vi "4.0.0_Airwatts_Tunings_&_Performance_Test_Max_Power_MODE.vi"(7 "Data in":T1, 8 "error in (no error)":errorcluster, 9 "AllControls In":T2, 10 "?":T3, 11 "Message Queue out":T4) -> (0 "error out":errorcluster, 1 "Flow":string, 2 "Data":T3, 3 "Message Queue Out":T4, 5 "Data out":T1)   [LabVIEW 2017]
uses:
  Depends/AMC/subVIs/TypeDefs/amc_Message Queue.ctl
  Depends/AMC/subVIs/TypeDefs/amc_Message.ctl
  Depends/Tools/Keyed Array/Tools_KeyedArray KeyedArray.ctl
  Ctrls/Data.ctl
  Ctrls/AllControls.ctl
  Ctrls/CSV_Data.ctl
  DIPC 692 Daemon API/typdef/get_parameter.ctl
  DIPC 692 Daemon API/typdef/calibration.ctl
  <vilib>/Analysis/baseanly.llb/Mean (DBL).vi
  Ctrls/AlarmIndex.ctl
  <vilib>/Analysis/NI_AALBase.lvlib
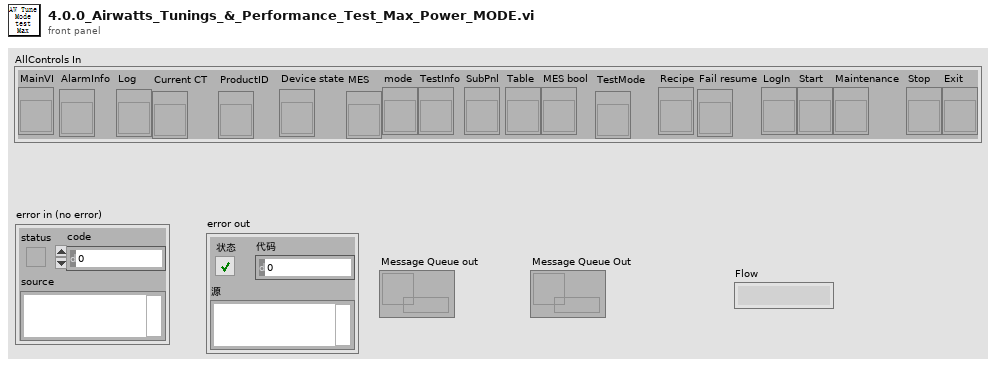
[diagram p1: front panel]
types:
  T1 = typedef "CSV_Data.ctl" = cluster{"Initialisation":cluster{"LMT - Connect UUT (con COM)":string, "LMT - Software Version (rrel)":string, "LMT - Write SKU file (wskuc)":string, "LMT - SKU file name":string, "Connect UUT DDM":string, "Read DDM EOL Timestamp - Mode":string, "Read DDM EOL Timestamp - Timestamp":string, "Read DDM EOL Timestamp - Rig ID":string, "Read DDM EOL Timestamp - Passmark ID":string, "Read DDM EOL Timestamp - Passmark Rev":string, "Software Version before flashing":string, "Read Hardware Serial":string, "UUT DDM SN":string, "Compare DDM SN with MES SN":string, "Backup PCBA Calibration EEPROM Response - CAL":string, "Flash Firmware Version":string, "Check SW Version":string, "Read DDM SW Version after flashing":string, "Set SKU Config":string, "Ready Status":string, "Set Device Mode to EOL":string, "DDM Parameter - Voltage":string, "DDM Parameter - Current":string, "DDM Parameter - Power":string, "DDM Parameter - Speed":string, "DDM Parameter - Pressure":string, "Tester Parameter - Voltage":string, "Tester Parameter - Current":string, "Tester Parameter - Power":string, "Tester Parameter - Ambient Pressure":string, "Tester Parameter - Ambient Temperature":string, "Calculated Parameter - DDM Pressure Corrected":string, "Calculated Parameter - DDM Real Power":string, "Calculated Parameter - Delta V":string}, "BEMF_Calibration":cluster{"Calibration Result - eol_cold_bemf_temp":string, "DDM Ambient Temp":string, "Restriction Plate Diameter":string, "Calibration Result - eol_bemf_mp_cold_coef_a":string, "Calibration Result - eol_bemf_mp_cold_coef_b":string, "Calibration Result - eol_bemf_mp_cold_coef_c":string, "Calibration Result - eol_bemf_lsi_cold_ref_coeffs":string, "Get - Calibration Result - eol_bemf_lsi_speed":string, "Get - Calibration Result - eol_bemf_lsi_integral_0":string, "Calibration Result - eol_bemf_lsi_integral_1":string, "Get - Calibration Result - eol_bemf_lsi_integral_2":string, "Get - Calibration Result - eol_cold_bemf":string, "Get - Calibration Result - eol_cold_bemf_fisf":string, "Finalise Calibration":string, "Compare -Calibration Result - eol_cold_bemf":string, "Compare -Calibration Result - eol_cold_bemf_fisf":string}, "ECO":cluster{"Reset Power Tune":string, "Reset BEMF FISF Calibration":string, "Restriction Plate Diameter":string, "ECO - Stabilisation Time":string, "ECO - DDM Parameter - Voltage":string, "ECO - DDM Parameter - Current":string, "ECO - DDM Parameter - Power":string, "ECO - DDM Parameter - Measured Power":string, "ECO - DDM Parameter - Speed":string, "ECO - DDM Parameter - Pressure":string, "ECO - Tester Parameter - Voltage":string, "ECO - Tester Parameter - Current":string, "ECO - Tester Parameter - Power":string, "ECO - Tester Parameter - Ambient Pressure":string, "ECO - Tester Parameter - Ambient Temperature":string, "ECO - Tester Parameter - Ambient Humidity":string, "ECO - Calculated Parameter - DDM Pressure Corrected":string, "ECO - Calculated Parameter - DDM Real Power":string, "ECO - Calculated Parameter - Delta V":string, "ECO - Calculated Parameter - Flowrate":string, "ECO - Calculated Parameter - Airwatt":string, "ECO - Formula":string, "PT ECO - Power Tune Mode Status":string}, "BOOST":cluster{"Restriction Plate Diameter":string, "BOOST - Stabilisation Time":string, "BOOST - DDM Parameter - Voltage":string, "BOOST - DDM Parameter - Current":string, "BOOST - DDM Parameter - Power":string, "BOOST - DDM Parameter - Measured Power":string, "BOOST - DDM Parameter - Speed":string, "BOOST - DDM Parameter - Pressure":string, "BOOST - Tester Parameter - Voltage":string, "BOOST - Tester Parameter - Current":string, "BOOST - Tester Parameter - Power":string, "BOOST - Tester Parameter - Ambient Pressure":string, "BOOST - Tester Parameter - Ambient Temperature":string, "BOOST - Tester Parameter - Ambient Humidity":string, "BOOST - Calculated Parameter - DDM Pressure Corrected":string, "BOOST - Calculated Parameter - DDM Real Power":string, "BOOST - Calculated Parameter - Delta V":string, "BOOST - Calculated Parameter - Flowrate":string, "BOOST - Calculated Parameter - Airwatt":string, "BOOST - Get AM Presence":string, "Air Muscle Turn Off Status":string, "BOOST - Air Muscle Calculated Parameter - Airwatt B":string, "BOOST - Air Muscle Calculate Airwatt Delta":string, "PT BOOST - Power Tune Mode Status":string, "Finalise Calibration":string, "ECO - Get AW Calibration value":string, "BOOST - Get AW Calibration value":string}, "MAX":cluster{"Restriction Plate Diameter":string, "MAX - Stabilisation Time":string, "Get Average Delta Tmag (LSIdelta_FISFdelta_LSItmag_FISFtmag_IIRtmag)":string, "Get Average Delta Tmag FISF":string, "MAX - DDM Parameter - Voltage":string, "MAX - DDM Parameter - Current":string, "MAX - DDM Parameter - Power":string, "MAX - DDM Parameter - Measured Power":string, "MAX - DDM Parameter - Speed":string, "MAX - DDM Parameter - Pressure":string, "MAX - Tester Parameter - Voltage":string, "MAX - Tester Parameter - Current":string, "MAX - Tester Parameter - Power":string, "MAX - Tester Parameter - Ambient Pressure":string, "MAX - Tester Parameter - Ambient Temperature":string, "MAX - Tester Parameter - Ambient Humidity":string, "MAX - Calculated Parameter - DDM Pressure Corrected":string, "MAX - Calculated Parameter - DDM Real Power":string, "MAX - Calculated Parameter - Delta V":string, "MAX - Calculated Parameter - Flowrate":string, "MAX - Calculated Parameter - Airwatt":string, "MAX_FISF_Check_Average_Delta_Tmag":string, "MAX - FISF - BEMF Finetune Result":string, "MAX tune - Delta P1":string, "MAX tune - Calculated Parameter - Airwatt":string, "Calculate Delta Airwatts - MAX finetune - Delta P2":string, "MAX finetune - DDM Parameter - Voltage":string, "MAX finetune - DDM Parameter - Current":string, "MAX finetune - DDM Parameter - Power":string, "MAX finetune - DDM Parameter - Measured Power":string, "MAX finetune - DDM Parameter - Speed":string, "MAX finetune - DDM Parameter - Pressure":string, "MAX finetune - Tester Parameter - Voltage":string, "MAX finetune - Tester Parameter - Current":string, "MAX finetune - Tester Parameter - Power":string, "MAX finetune - Tester Parameter - Ambient Pressure":string, "MAX finetune - Tester Parameter - Ambient Temperature":string, "MAX finetune - Tester Parameter - Ambient Humidity":string, "MAX finetune - Calculated Parameter - DDM Pressure Corrected":string, "MAX finetune - Calculated Parameter - DDM Real Power":string, "MAX finetune - Calculated Parameter - Delta V":string, "MAX finetune - Calculated Parameter - Flowrate":string, "MAX finetune - Calculated Parameter - Airwatt":string, "Check Derate Result":string, "Delta Tmag FISF":string, "Get Hot BEMF Result":string, "Calculate delta Pressure":string, "Finalise Calibration":string, "Calculate & Check Delta BEMF":string, "Delta P Airwatts Value":string}, "LL":cluster{"DDM Ambient Temp":string, "Restriction Plate Diameter":string, "LL - DDM Parameter - Voltage":string, "LL - DDM Parameter - Current":string, "LL - DDM Parameter - Power":string, "LL - DDM Parameter - Measured Power":string, "LL - DDM Parameter - Speed":string, "LL - DDM Parameter - Pressure":string, "LL - Tester Parameter - Voltage":string, "LL - Tester Parameter - Current":string, "LL - Tester Parameter - Power":string, "LL - DDM Real Power":string, "LL - Calibrate Task Detect LL":string}, "HL":cluster{"HL - DDM Parameter - Voltage":string, "HL - DDM Parameter - Current":string, "HL - DDM Parameter - Power":string, "HL - DDM Parameter - Measured Power":string, "HL - DDM Parameter - Speed":string, "HL - DDM Parameter - Pressure":string, "HL - Tester Parameter - Voltage":string, "HL - Tester Parameter - Current":string, "HL - Tester Parameter - Power":string, "HL - DDM Real Power":string, "HL - Calibrate Task Detect HL":string}, "LH":cluster{"Restriction Plate Diameter":string, "LH - DDM Parameter - Voltage":string, "LH - DDM Parameter - Current":string, "LH - DDM Parameter - Power":string, "LH - DDM Parameter - Measured Power":string, "LH - DDM Parameter - Speed":string, "LH - DDM Parameter - Pressure":string, "LH - Tester Parameter - Voltage":string, "LH - Tester Parameter - Current":string, "LH - Tester Parameter - Power":string, "LH - DDM Real Power":string, "LH - Calibrate Task Detect LH":string}, "HH":cluster{"HH - DDM Parameter - Voltage":string, "HH - DDM Parameter - Current":string, "HH - DDM Parameter - Power":string, "HH - DDM Parameter - Measured Power":string, "HH - DDM Parameter - Speed":string, "HH - DDM Parameter - Pressure":string, "HH - Tester Parameter - Voltage":string, "HH - Tester Parameter - Current":string, "HH - Tester Parameter - Power":string, "HH - DDM Real Power":string, "HH - Calibrate Task Detect HH":string}, "Inlet Blockage Calibration":cluster{"Inlet Blockage Calibration - DDM Parameter - Voltage":string, "Inlet Blockage Calibration - DDM Parameter - Current":string, "Inlet Blockage Calibration - DDM Parameter - Power":string, "Inlet Blockage Calibration - DDM Parameter - Measured Power":string, "Inlet Blockage Calibration - DDM Parameter - Speed":string, "Inlet Blockage Calibration - DDM Parameter - Pressure":string, "Inlet Blockage Calibration - Tester Parameter - Voltage":string, "Inlet Blockage Calibration - Tester Parameter - Current":string, "Inlet Blockage Calibration - Tester Parameter - Power":string, "Inlet Blockage Calibration - DDM Real Power":string, "Calibration Inlet Blockage_E":string, "Finalise Calibration":string, "Get Task Detect LL":string, "Get Task Detect HL":string, "Get Task Detect LH":string, "Get Task Detect HH":string, "Calibration Inlet Blockage":string, "Calibration eol cold bemf temp":string}, "GOOD":cluster{"GOOD UNIT - Clear EEPROM Error Log":string, "GOOD UNIT - Write Product Timestamp - Mode":string, "GOOD UNIT - Write Product Timestamp - Timestamp":string, "GOOD UNIT - Write Product Timestamp - Rig ID":string, "GOOD UNIT - Write Product Timestamp - Passmark ID":string, "GOOD UNIT - Write Product Timestamp - Passmark Rev":string, "GOOD UNIT - Set Device Mode to PROD":string, "GOOD UNIT - Backup PCBA Calibration EEPROM Response":string, "GOOD UNIT - Check Security Bit":string, "GOOD UNIT - Set Calibration Lock":string, "GOOD UNIT - Get_Calibration_Lock":string, "GOOD UNIT - Disconnect UUT":string}, "NG":cluster{"NG UNIT - Read NVM Error":string, "NG UNIT - Set Device Mode to FCT":string, "NG UNIT - Backup PCBA Calibration EEPROM Response - CAL":string, "NG UNIT - Backup PCBA Calibration EEPROM Response - ERROR":string, "NG UNIT - Backup PCBA Calibration EEPROM Response - USAGE":string, "NG UNIT - Disconnect UUT":string}, "SN":string, "Table":string[][], "Count":cluster{"Total":i32, "OK":i32, "NG":i32, "Yield":dbl}, "Start Time":timestamp, "daemon reference":refnum<k5>, "CT":dbl, "Config":string[][], "OK/NG":bool, "Station ID":string, "MES DDM SN":string, "MES PCBA SN":string, "Retest":string, "Lux":string, "Initialisation_Status":cluster{"LMT - Connect UUT (con COM)":string, "LMT - Software Version (rrel)":string, "LMT - Write SKU file (wskuc)":string, "LMT - SKU file name":string, "Connect UUT DDM":string, "Read DDM EOL Timestamp - Mode":string, "Read DDM EOL Timestamp - Timestamp":string, "Read DDM EOL Timestamp - Rig ID":string, "Read DDM EOL Timestamp - Passmark ID":string, "Read DDM EOL Timestamp - Passmark Rev":string, "Software Version before flashing":string, "Read Hardware Serial":string, "UUT DDM SN":string, "Compare DDM SN with MES SN":string, "Backup PCBA Calibration EEPROM Response - CAL":string, "Flash Firmware Version":string, "Check SW Version":string, "Read DDM SW Version after flashing":string, "Set SKU Config":string, "Ready Status":string, "Set Device Mode to EOL":string, "DDM Parameter - Voltage":string, "DDM Parameter - Current":string, "DDM Parameter - Power":string, "DDM Parameter - Speed":string, "DDM Parameter - Pressure":string, "Tester Parameter - Voltage":string, "Tester Parameter - Current":string, "Tester Parameter - Power":string, "Tester Parameter - Ambient Pressure":string, "Tester Parameter - Ambient Temperature":string, "Calculated Parameter - DDM Pressure Corrected":string, "Calculated Parameter - DDM Real Power":string, "Calculated Parameter - Delta V":string}, "BEMF_Calibration_Status":cluster{"Calibration Result - eol_cold_bemf_temp":string, "DDM Ambient Temp":string, "Restriction Plate Diameter":string, "Calibration Result - eol_bemf_mp_cold_coef_a":string, "Calibration Result - eol_bemf_mp_cold_coef_b":string, "Calibration Result - eol_bemf_mp_cold_coef_c":string, "Calibration Result - eol_bemf_lsi_cold_ref_coeffs":string, "Get - Calibration Result - eol_bemf_lsi_speed":string, "Get - Calibration Result - eol_bemf_lsi_integral_0":string, "Calibration Result - eol_bemf_lsi_integral_1":string, "Get - Calibration Result - eol_bemf_lsi_integral_2":string, "Get - Calibration Result - eol_cold_bemf":string, "Get - Calibration Result - eol_cold_bemf_fisf":string, "Finalise Calibration":string, "Compare -Calibration Result - eol_cold_bemf":string, "Compare -Calibration Result - eol_cold_bemf_fisf":string}, "ECO_Status":cluster{"Reset Power Tune":string, "Reset BEMF FISF Calibration":string, "Restriction Plate Diameter":string, "ECO - Stabilisation Time":string, "ECO - DDM Parameter - Voltage":string, "ECO - DDM Parameter - Current":string, "ECO - DDM Parameter - Power":string, "ECO - DDM Parameter - Measured Power":string, "ECO - DDM Parameter - Speed":string, "ECO - DDM Parameter - Pressure":string, "ECO - Tester Parameter - Voltage":string, "ECO - Tester Parameter - Current":string, "ECO - Tester Parameter - Power":string, "ECO - Tester Parameter - Ambient Pressure":string, "ECO - Tester Parameter - Ambient Temperature":string, "ECO - Tester Parameter - Ambient Humidity":string, "ECO - Calculated Parameter - DDM Pressure Corrected":string, "ECO - Calculated Parameter - DDM Real Power":string, "ECO - Calculated Parameter - Delta V":string, "ECO - Calculated Parameter - Flowrate":string, "ECO - Calculated Parameter - Airwatt":string, "ECO - Formula":string, "PT ECO - Power Tune Mode Status":string}, "BOOST_Status":cluster{"Restriction Plate Diameter":string, "BOOST - Stabilisation Time":string, "BOOST - DDM Parameter - Voltage":string, "BOOST - DDM Parameter - Current":string, "BOOST - DDM Parameter - Power":string, "BOOST - DDM Parameter - Measured Power":string, "BOOST - DDM Parameter - Speed":string, "BOOST - DDM Parameter - Pressure":string, "BOOST - Tester Parameter - Voltage":string, "BOOST - Tester Parameter - Current":string, "BOOST - Tester Parameter - Power":string, "BOOST - Tester Parameter - Ambient Pressure":string, "BOOST - Tester Parameter - Ambient Temperature":string, "BOOST - Tester Parameter - Ambient Humidity":string, "BOOST - Calculated Parameter - DDM Pressure Corrected":string, "BOOST - Calculated Parameter - DDM Real Power":string, "BOOST - Calculated Parameter - Delta V":string, "BOOST - Calculated Parameter - Flowrate":string, "BOOST - Calculated Parameter - Airwatt":string, "BOOST - Get AM Presence":string, "Air Muscle Turn Off Status":string, "BOOST - Air Muscle Calculated Parameter - Airwatt B":string, "BOOST - Air Muscle Calculate Airwatt Delta":string, "PT BOOST - Power Tune Mode Status":string, "Finalise Calibration":string, "ECO - Get AW Calibration value":string, "BOOST - Get AW Calibration value":string}, "MAX_Status":cluster{"Restriction Plate Diameter":string, "MAX - Stabilisation Time":string, "Get Average Delta Tmag (LSIdelta_FISFdelta_LSItmag_FISFtmag_IIRtmag)":string, "Get Average Delta Tmag FISF":string, "MAX - DDM Parameter - Voltage":string, "MAX - DDM Parameter - Current":string, "MAX - DDM Parameter - Power":string, "MAX - DDM Parameter - Measured Power":string, "MAX - DDM Parameter - Speed":string, "MAX - DDM Parameter - Pressure":string, "MAX - Tester Parameter - Voltage":string, "MAX - Tester Parameter - Current":string, "MAX - Tester Parameter - Power":string, "MAX - Tester Parameter - Ambient Pressure":string, "MAX - Tester Parameter - Ambient Temperature":string, "MAX - Tester Parameter - Ambient Humidity":string, "MAX - Calculated Parameter - DDM Pressure Corrected":string, "MAX - Calculated Parameter - DDM Real Power":string, "MAX - Calculated Parameter - Delta V":string, "MAX - Calculated Parameter - Flowrate":string, "MAX - Calculated Parameter - Airwatt":string, "MAX_FISF_Check_Average_Delta_Tmag":string, "MAX - FISF - BEMF Finetune Result":string, "MAX tune - Delta P1":string, "MAX tune - Calculated Parameter - Airwatt":string, "Calculate Delta Airwatts - MAX finetune - Delta P2":string, "MAX finetune - DDM Parameter - Voltage":string, "MAX finetune - DDM Parameter - Current":string, "MAX finetune - DDM Parameter - Power":string, "MAX finetune - DDM Parameter - Measured Power":string, "MAX finetune - DDM Parameter - Speed":string, "MAX finetune - DDM Parameter - Pressure":string, "MAX finetune - Tester Parameter - Voltage":string, "MAX finetune - Tester Parameter - Current":string, "MAX finetune - Tester Parameter - Power":string, "MAX finetune - Tester Parameter - Ambient Pressure":string, "MAX finetune - Tester Parameter - Ambient Temperature":string, "MAX finetune - Tester Parameter - Ambient Humidity":string, "MAX finetune - Calculated Parameter - DDM Pressure Corrected":string, "MAX finetune - Calculated Parameter - DDM Real Power":string, "MAX finetune - Calculated Parameter - Delta V":string, "MAX finetune - Calculated Parameter - Flowrate":string, "MAX finetune - Calculated Parameter - Airwatt":string, "Check Derate Result":string, "Delta Tmag FISF":string, "Get Hot BEMF Result":string, "Calculate delta Pressure":string, "Finalise Calibration":string, "Calculate & Check Delta BEMF":string, "Delta P Airwatts Value":string}, "LL_Status":cluster{"DDM Ambient Temp":string, "Restriction Plate Diameter":string, "LL - DDM Parameter - Voltage":string, "LL - DDM Parameter - Current":string, "LL - DDM Parameter - Power":string, "LL - DDM Parameter - Measured Power":string, "LL - DDM Parameter - Speed":string, "LL - DDM Parameter - Pressure":string, "LL - Tester Parameter - Voltage":string, "LL - Tester Parameter - Current":string, "LL - Tester Parameter - Power":string, "LL - DDM Real Power":string, "LL - Calibrate Task Detect LL":string}, "HL_Status":cluster{"HL - DDM Parameter - Voltage":string, "HL - DDM Parameter - Current":string, "HL - DDM Parameter - Power":string, "HL - DDM Parameter - Measured Power":string, "HL - DDM Parameter - Speed":string, "HL - DDM Parameter - Pressure":string, "HL - Tester Parameter - Voltage":string, "HL - Tester Parameter - Current":string, "HL - Tester Parameter - Power":string, "HL - DDM Real Power":string, "HL - Calibrate Task Detect HL":string}, "LH_Status":cluster{"Restriction Plate Diameter":string, "LH - DDM Parameter - Voltage":string, "LH - DDM Parameter - Current":string, "LH - DDM Parameter - Power":string, "LH - DDM Parameter - Measured Power":string, "LH - DDM Parameter - Speed":string, "LH - DDM Parameter - Pressure":string, "LH - Tester Parameter - Voltage":string, "LH - Tester Parameter - Current":string, "LH - Tester Parameter - Power":string, "LH - DDM Real Power":string, "LH - Calibrate Task Detect LH":string}, "HH_Status":cluster{"HH - DDM Parameter - Voltage":string, "HH - DDM Parameter - Current":string, "HH - DDM Parameter - Power":string, "HH - DDM Parameter - Measured Power":string, "HH - DDM Parameter - Speed":string, "HH - DDM Parameter - Pressure":string, "HH - Tester Parameter - Voltage":string, "HH - Tester Parameter - Current":string, "HH - Tester Parameter - Power":string, "HH - DDM Real Power":string, "HH - Calibrate Task Detect HH":string}, "Inlet Blockage Calibration_Status":cluster{"Inlet Blockage Calibration - DDM Parameter - Voltage":string, "Inlet Blockage Calibration - DDM Parameter - Current":string, "Inlet Blockage Calibration - DDM Parameter - Power":string, "Inlet Blockage Calibration - DDM Parameter - Measured Power":string, "Inlet Blockage Calibration - DDM Parameter - Speed":string, "Inlet Blockage Calibration - DDM Parameter - Pressure":string, "Inlet Blockage Calibration - Tester Parameter - Voltage":string, "Inlet Blockage Calibration - Tester Parameter - Current":string, "Inlet Blockage Calibration - Tester Parameter - Power":string, "Inlet Blockage Calibration - DDM Real Power":string, "Calibration Inlet Blockage_E":string, "Finalise Calibration":string, "Get Task Detect LL":string, "Get Task Detect HL":string, "Get Task Detect LH":string, "Get Task Detect HH":string, "Calibration Inlet Blockage":string, "Calibration eol cold bemf temp":string}, "GOOD_Status":cluster{"GOOD UNIT - Clear EEPROM Error Log":string, "GOOD UNIT - Write Product Timestamp - Mode":string, "GOOD UNIT - Write Product Timestamp - Timestamp":string, "GOOD UNIT - Write Product Timestamp - Rig ID":string, "GOOD UNIT - Write Product Timestamp - Passmark ID":string, "GOOD UNIT - Write Product Timestamp - Passmark Rev":string, "GOOD UNIT - Set Device Mode to PROD":string, "GOOD UNIT - Backup PCBA Calibration EEPROM Response":string, "GOOD UNIT - Check Security Bit":string, "GOOD UNIT - Set Calibration Lock":string, "GOOD UNIT - Get_Calibration_Lock":string, "GOOD UNIT - Disconnect UUT":string}, "NG_Status":cluster{"NG UNIT - Read NVM Error":string, "NG UNIT - Set Device Mode to FCT":string, "NG UNIT - Backup PCBA Calibration EEPROM Response - CAL":string, "NG UNIT - Backup PCBA Calibration EEPROM Response - ERROR":string, "NG UNIT - Backup PCBA Calibration EEPROM Response - USAGE":string, "NG UNIT - Disconnect UUT":string}, "SKU":string, "Plate_Diameter":string, "Alarm":string}
  T2 = typedef "AllControls.ctl" = cluster{"MainVI":refnum<vi>, "AlarmInfo":refnum<vi>, "Log":refnum<vi>, "Current CT":refnum<vi>, "ProductID":refnum<vi>, "Device state":refnum<vi>, "MES":refnum<vi>, "mode":refnum<vi>, "TestInfo":refnum<vi>, "SubPnl":refnum<vi>, "Table":refnum<vi>, "MES bool":refnum<vi>, "TestMode":refnum<vi>, "Recipe":refnum<vi>, "Fail resume":refnum<vi>, "LogIn":refnum<vi>, "Start":refnum<vi>, "Maintenance":refnum<vi>, "Stop":refnum<vi>, "Exit":refnum<vi>}
  T3 = typedef "Data.ctl" = cluster{"Initialisation":cluster{"DDM_Parameter":dbl[], "DDM_Parameter_status":bool[], "Get_Tester_Parameter":dbl[], "Get_Tester_Parameter_status":bool[], "Cal_Tester_Parameter":dbl[], "Cal_Tester_Parameter_status":bool[], "sw_version_before_status":bool, "sw_version_after_status":bool, "Set_SKU_Config_With_LMT_status":bool, "FCT_timestamp_status":bool, "LMT_Connect_to_UUT_status":bool}, "BEMF_Calibration":cluster{"Read_ambient_temperature":dbl, "Calibration_Vaule":dbl[], "Calibration_Vaule _B":dbl[], "Calibration_Vaule_status":bool[], "Calibration_Vaule_B_status":bool[]}, "ECO":cluster{"DDM_Parameter":dbl[], "DDM_Parameter_status":bool[], "Get_Tester_Parameter":dbl[], "Get_Tester_Parameter_status":bool[], "Cal_Tester_Parameter":dbl[], "Cal_Tester_Parameter_status":bool[], "DDM_Parameter_after_power_tune":dbl[], "Get_Tester_Parameter_after_power_tune":dbl[], "Cal_Tester_Parameter_after_power_tune":dbl[], "Cal_Tester_Parameter_after_power_tune_status":bool[], "Delta_P":dbl}, "BOOST":cluster{"DDM_Parameter":dbl[], "DDM_Parameter_status":bool[], "Get_Tester_Parameter":dbl[], "Get_Tester_Parameter_status":bool[], "Cal_Tester_Parameter":dbl[], "Cal_Tester_Parameter_status":bool[], "DDM_Parameter_after_power_tune":dbl[], "Get_Tester_Parameter_after_power_tune":dbl[], "Cal_Tester_Parameter_after_power_tune":dbl[], "Cal_Tester_Parameter_after_power_tune_status":bool[], "airwatts_am_off":dbl, "AW_Delta_(AM_on_and_off)":dbl, "AW_Delta_(AM_on_and_off)_Status":bool, "Delta_P":dbl}, "MAX":cluster{"Average_Tmag_Data":cluster{"LSI Delta in degC":dbl, "FISF Delta in degc":dbl, "LSI Tmag in degC":dbl, "Fisf Tmag in degC":dbl, "IIR Tmag in degC":dbl}, "DDM_Parameter":dbl[], "DDM_Parameter_status":bool[], "Get_Tester_Parameter":dbl[], "Get_Tester_Parameter_status":bool[], "Cal_Tester_Parameter":dbl[], "BEMF_Finetune":cluster{"eol_bemf_mp_cold_coef_c":dbl, "eol_cold_bemf_fisf_offset":dbl}, "AW_Tune":cluster{"delta_P1":dbl, "delta_P_Setting":dbl}, "DDM_Parameter_after_Airwatts_Tune":dbl[], "Get_Tester_Parameter_after_Airwatts_Tune":dbl[], "Cal_Tester_Parameter_after_Airwatts_Tune":dbl[], "DDM_Parameter_after_Airwatts_Finetune":dbl[], "Get_Tester_Parameter_after_Airwatts_Finetune":dbl[], "Cal_Tester_Parameter_after_Airwatts_Finetune":dbl[], "AW_Finetune":cluster{"delta_P2":dbl, "delta_P_Setting":dbl}, "Delta_Tmag_after_tune":cluster{"LSI Delta in degC":dbl, "FISF Delta in degc":dbl, "LSI Tmag in degC":dbl, "Fisf Tmag in degC":dbl, "IIR Tmag in degC":dbl}, "Hot Bemf in mV":dbl, "DDM_Pressure":dbl, "Delta_Pressure":dbl, " Cold Bemf in mV":dbl, " delta Bemf":dbl, " delta p":dbl, "Delta_Pressure_status":bool, " delta Bemf_status":bool, "LSI Delta in degC_status":bool, "FISF Delta in degc_status":bool, "Max_check_derate_status_status":bool, "Average_All_data":dbl[][], "Average_Tmag_Data_status":bool[], "Average_Tmag_Data_after_tune_status":bool[], "Cal_Tester_Parameter_status":bool[], "Cal_Tester_Parameter_status_after_Airwatts_Tune":bool[], "Cal_Tester_Parameter_status_after_Airwatts_FineTune":bool[]}, "Task_Detect_Calib":cluster{"LL":cluster{"DDM_Parameter":dbl[], "DDM_Parameter_status":bool[], "Get_Tester_Parameter":dbl[], "Get_Tester_Parameter_status":bool[], "Set_task_detect_A":dbl, "Set_task_detect_A_Status":bool}, "HL":cluster{"DDM_Parameter":dbl[], "DDM_Parameter_status":bool[], "Get_Tester_Parameter":dbl[], "Get_Tester_Parameter_status":bool[], "Set_task_detect_B":dbl, "Set_task_detect_B_Status":bool}, "LH":cluster{"DDM_Parameter":dbl[], "DDM_Parameter_status":bool[], "Get_Tester_Parameter":dbl[], "Get_Tester_Parameter_status":bool[], "Set_task_detect_C":dbl, "Set_task_detect_C_Status":bool}, "HH":cluster{"DDM_Parameter":dbl[], "DDM_Parameter_status":bool[], "Get_Tester_Parameter":dbl[], "Get_Tester_Parameter_status":bool[], "Set_task_detect_D":dbl, "Read_and_check_calibration_Status":bool[], "Set_task_detect_D_Status":bool}, "Get_eol_inlet_blockage_E":dbl, "Calib_vaule":cluster{"Get_task_detect_LL":dbl, "Get_task_detect_HL":dbl, "Get_task_detect_LH":dbl, "Get_task_detect_HH":dbl, "eol_inlet_blockage":dbl, "eol_code_bemf_temp":dbl}, "calibrated temp":dbl, "Inlet_Blockage_Calibration":cluster{"DDM_Parameter":dbl[], "DDM_Parameter_status":bool[], "Get_Tester_Parameter":dbl[], "Get_Tester_Parameter_status":bool[]}, "Get_eol_inlet_blockage_E_Status":bool}, "good":cluster{"Write_Product_TS":cluster{"TIMESTAMP":i64, "RIG_ID":i64, "PASSMARK_ID":i64, "PASSMARK_REV":i64}, "Read_Product_TS":cluster{"TIMESTAMP":i64, "RIG_ID":i64, "PASSMARK_ID":i64, "PASSMARK_REV":i64}, "Good_Check_Secuity_Bit_Stauts":bool}}
  T4 = typedef "amc_Message Queue.ctl" = refnum<queue>
  T5 = typedef "HD Config.ctl" = cluster{" PC":cluster{"PC Address":u8[], "PC Port":i32}, "FCO":cluster{"COM":refnum<visa-resource-name>, "Baudrate":u32}, "DC Power ":cluster{"COM":refnum<visa-resource-name>, "Baudrate":u32}, "PW3336":cluster{"COM":refnum<visa-resource-name>, "Baudrate":u32}, "Lefoo":cluster{"COM":refnum<visa-resource-name>, "Baudrate":u32}, "Tempt&Hum":cluster{"COM":refnum<visa-resource-name>, "Baudrate":u32}, "DIPC":cluster{"COM":refnum<visa-resource-name>}, "Daemon":cluster{"IP Address":string, "Port":u16, "Retry":u16}, "Motor":cluster{"COM":refnum<visa-resource-name>, "Baudrate":u32}, "Fail_resume_mode":bool, "GRR":bool}
  T6 = typedef "AlarmIndex.ctl" = enum16{"E-Stop", "Safety light grid", "UUT Sealing Cylinder HomePoint", "UUT Sealing Cylinder WorkPoint", "Orifice fixed Cylinder L HomePoint", "Orifice fixed Cylinder L WorkPoint", "Orifice fixed Cylinder R HomePoint", "Orifice fixed Cylinder R WorkPoint", "UUT Cylinder HomePoint", "UUT Cylinder WorkPoint", "Carrier fixed Cylinder L HomePoint", "Carrier fixed Cylinder L WorkPoint", "Carrier fixed Cylinder R HomePoint", "Carrier fixed Cylinder R WorkPoint", "Probe Cylinder HomePoint", "Probe Cylinder WorkPoint", "Motor Error", "Test Error"}
  T7 = typedef "get_parameter.ctl" = string
  T8 = cluster{"LSI Delta in degC":dbl, "FISF Delta in degc":dbl, "LSI Tmag in degC":dbl, "Fisf Tmag in degC":dbl, "IIR Tmag in degC":dbl}
  T9 = cluster{"LSI Delta in degC":string, "FISF Delta in degc":string, "LSI Tmag in degC":string, "Fisf Tmag in degC":string, "IIR Tmag in degC":string}
  T10 = typedef "calibration.ctl" = string
  T11 = typedef "Position Config.ctl" = cluster{"OrificeSize_12.7":i32, "OrificeSize_13":i32, "OrificeSize_30":i32, "OrificeSize_16":i32}
  T12 = cluster{"[0]":dbl, "[1]":dbl, "[2]":dbl, "[3]":dbl, "[4]":dbl}
  T13 = typedef "airwatt tune parameter.ctl" = cluster{"Index(0-5)":i64, "Target power mW":i64, "Offset power mW":i64}
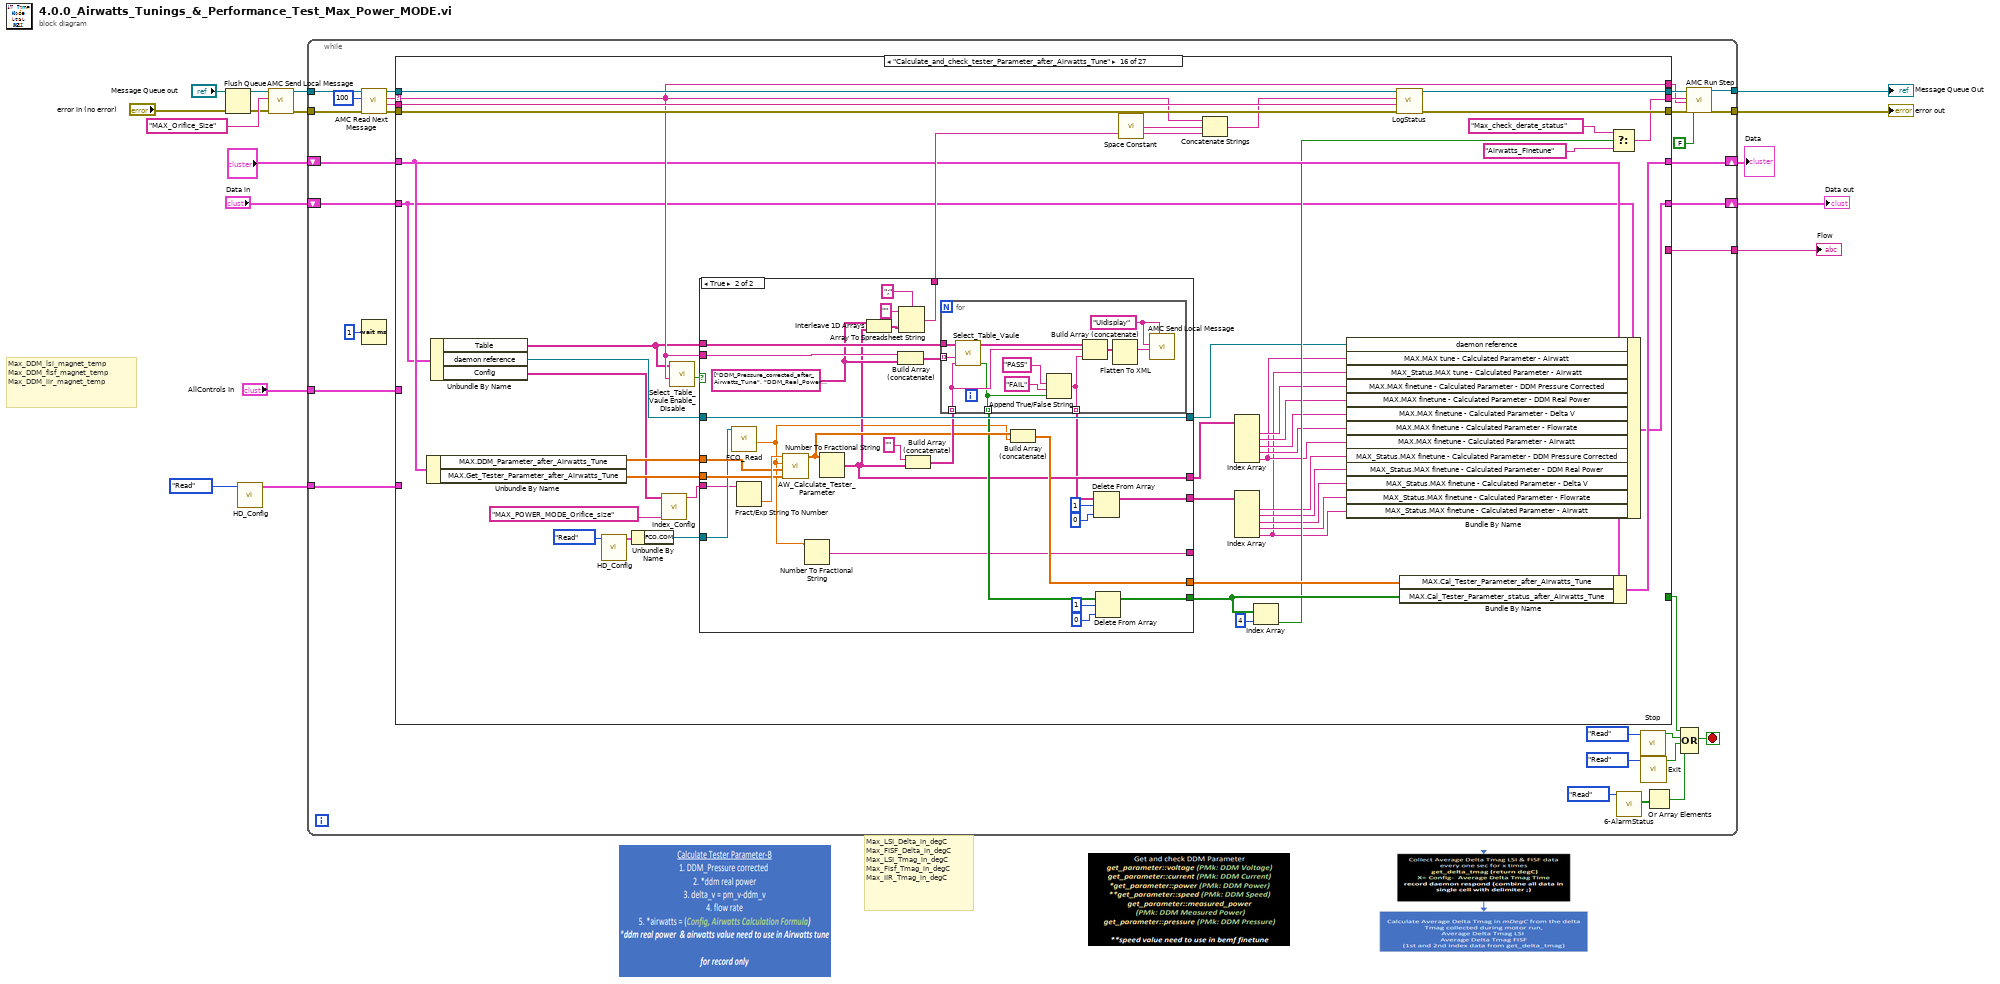
[diagram p0: block diagram]
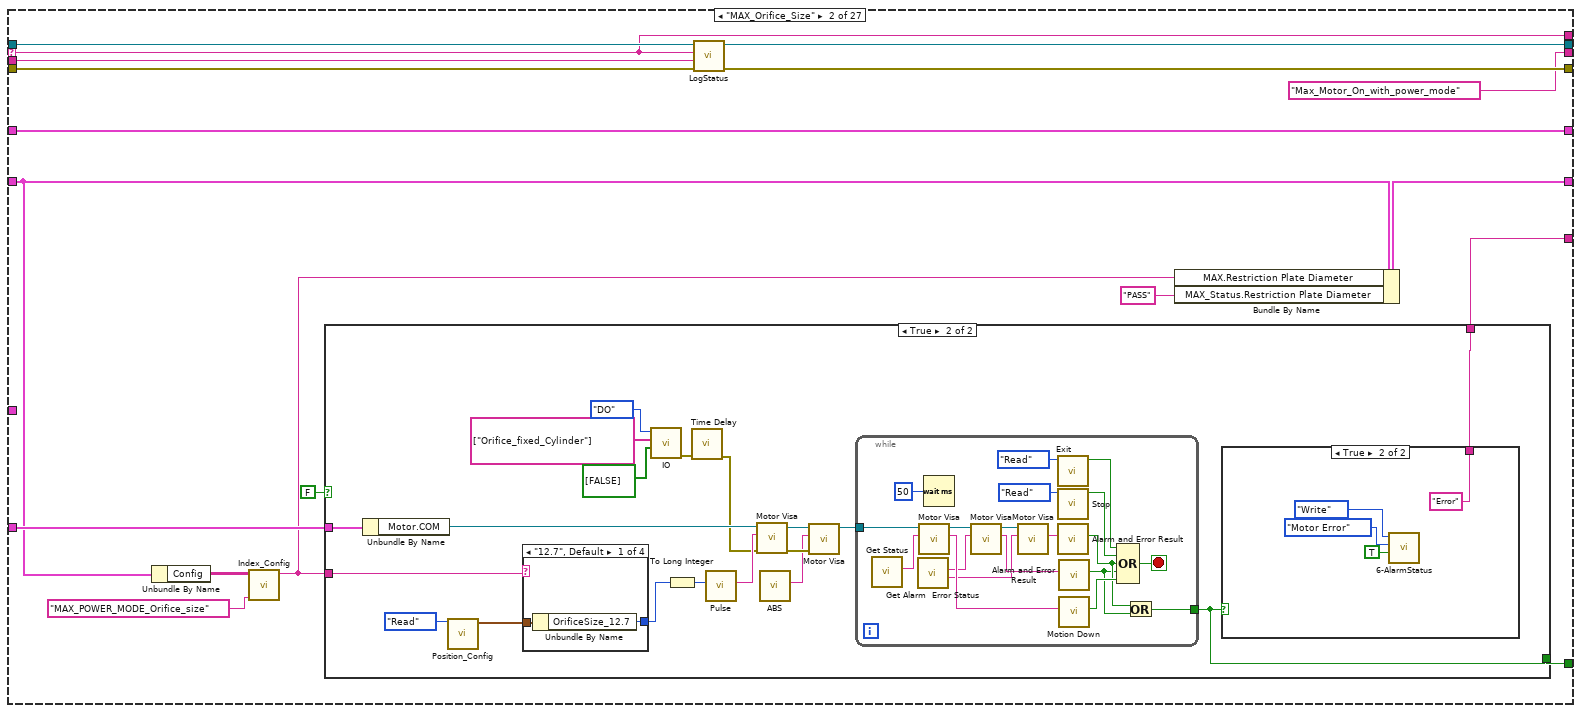
[diagram p3: hidden frame]
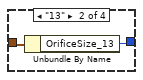
[diagram p5: hidden frame]
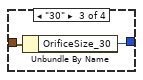
[diagram p6: hidden frame]
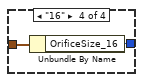
[diagram p7: hidden frame]
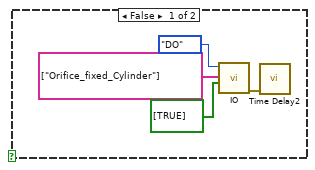
[diagram p8: hidden frame]
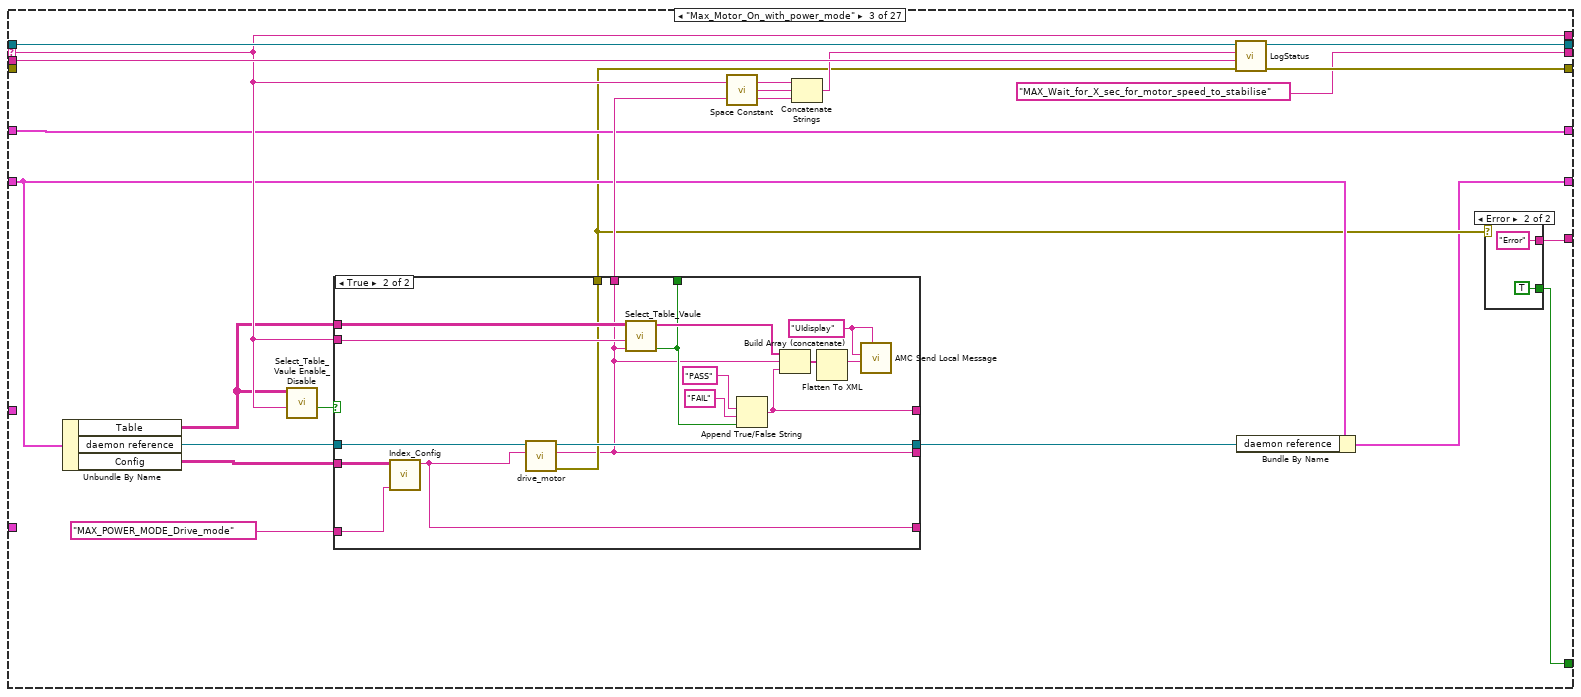
[diagram p9: hidden frame]
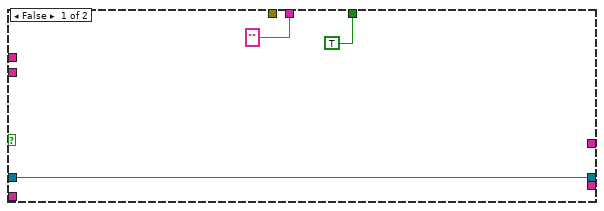
[diagram p11: hidden frame]
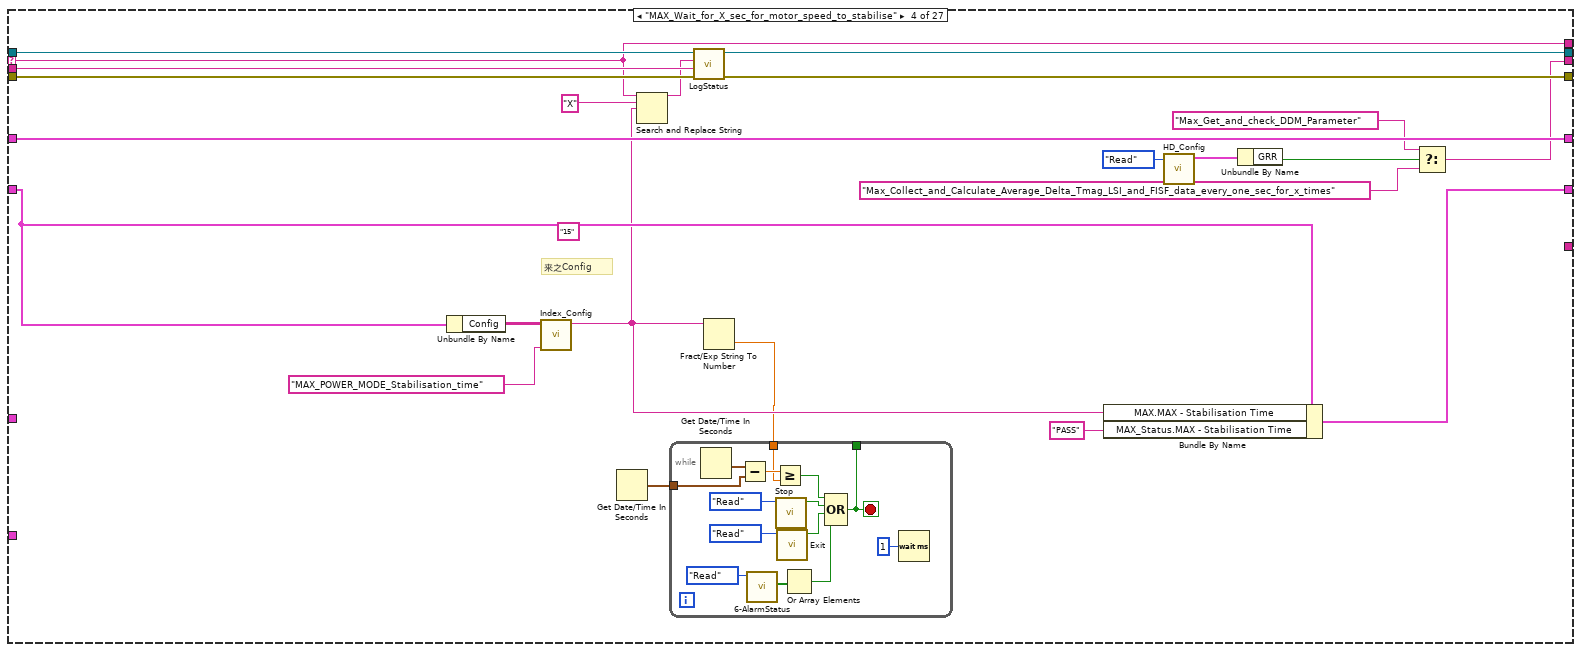
[diagram p12: hidden frame]
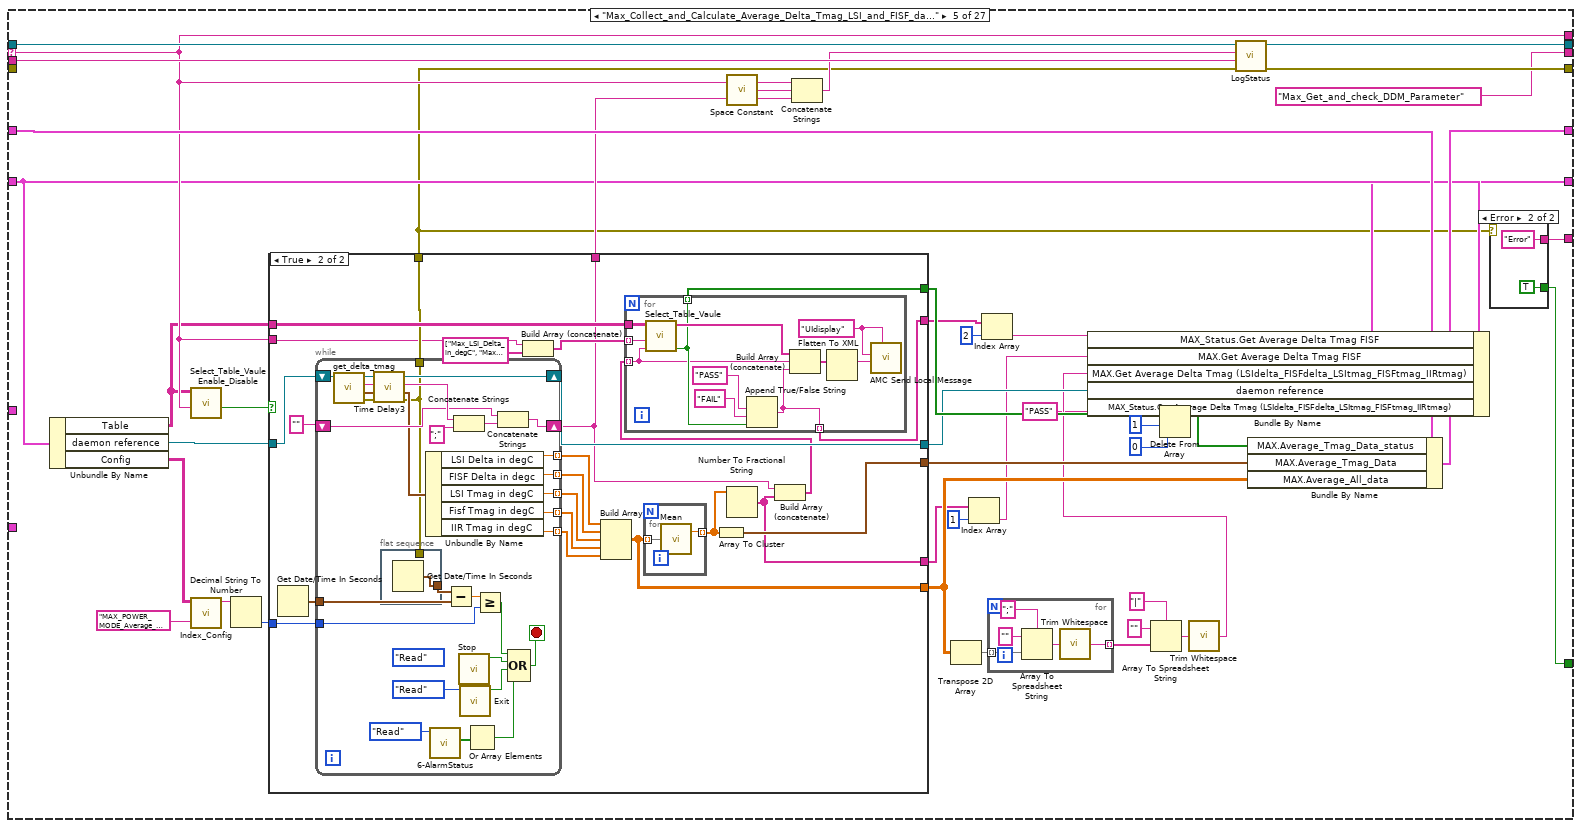
[diagram p13: hidden frame]
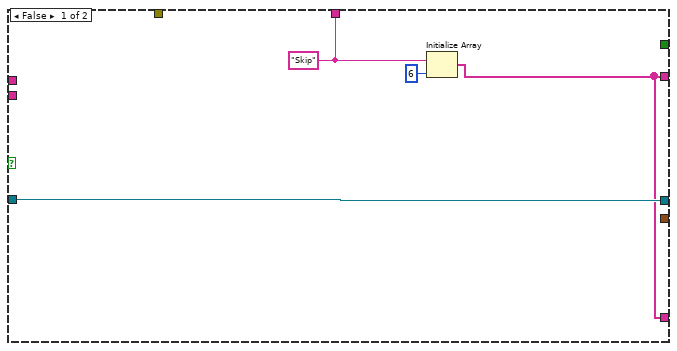
[diagram p15: hidden frame]
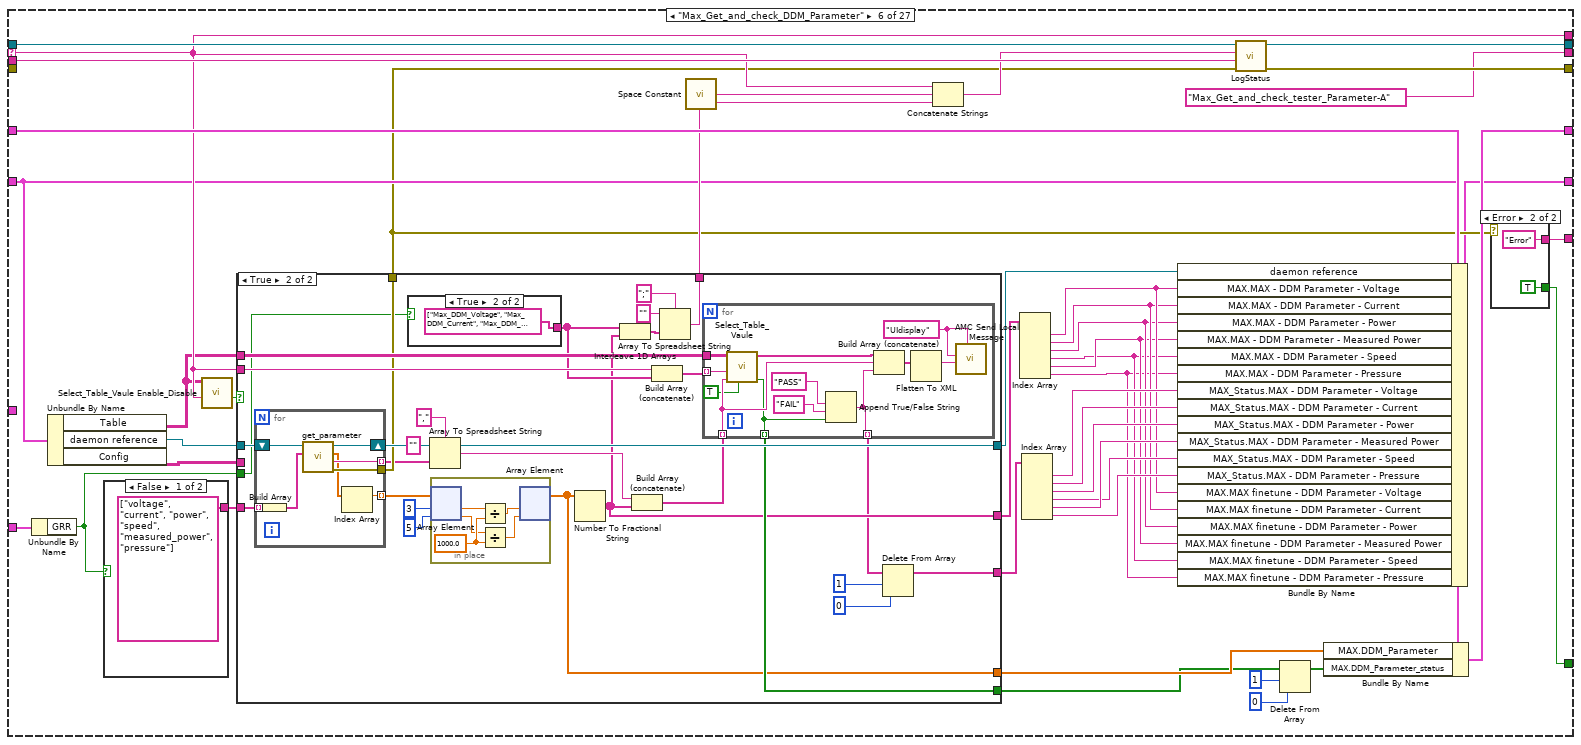
[diagram p16: hidden frame]
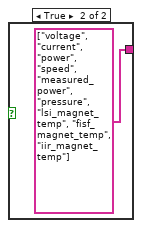
[diagram p17: hidden frame]
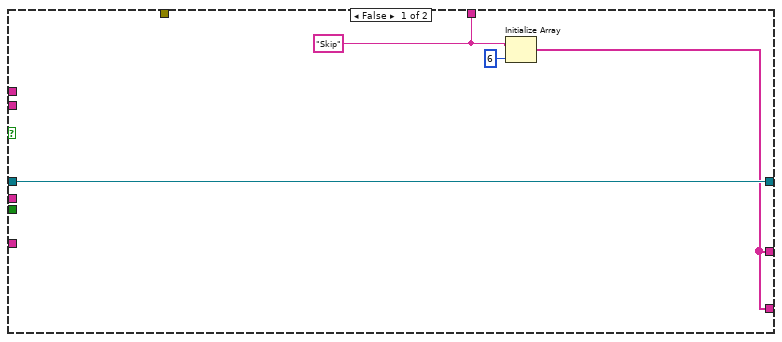
[diagram p19: hidden frame]
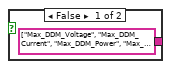
[diagram p20: hidden frame]
diagram:
  # "Max_DDM_lsi_magnet_temp\nMax_DDM_fisf_magnet_temp\nMax_DDM_iir_magnet_temp"
  # "Max_LSI_Delta_in_degC\nMax_FISF_Delta_in_degC\nMax_LSI_Tmag_in_degC\nMax_Fisf_Tmag_in_degC\nMax_IIR_Tmag_in_degC"
  n1 = Flush Queue(queue="Message Queue out") -> (queue out=w4:T4)  [unwired: 1 in, 2 out]
  n2 = call "HD_Config.vi"("Step"=enum16{"Initial", "Write", "Read"}."Read") -> ("HD Config out"=w8:T5)  [unwired: 9 in, 1 out]
  n3 = call "AMC Send Local Message.vi"("error in (no error)"="error in (no error)", "Message Name"="MAX_Orifice_Size", "Message Queue in"=w4) -> ("error out"=w13:errorcluster, "Message Queue out"=w14:T4)  [unwired: 7 in]
  n4 = while {
    tunnel: w14 -> [w47]
    tunnel: [w43] -> w6
    tunnel: w13 -> [w41]
    tunnel: [w38] -> w5
    shift-right: [w34] -> w10
    shift-left: "?" -> [w35]
    tunnel: w8 -> [w33]
    tunnel: [w29] -> w7
    shift-right: [w21] -> w1
    shift-left: "Data in" -> [w22]
    tunnel: "AllControls In" -> [w20]
    stop <- w23 stop-if-true
    n5 = call "AMC Read Next Message.vi"("error in (no error)"=w41, "timeout (1ms)"=100, "Message Queue in"=w47) -> ("error out"=w40:errorcluster, "Message Value"=w31:string, "Message Name"=w45:string, "Message Queue out"=w46:T4)  [unwired: 1 in, 4 out]
    n6 = Wait (ms)(milliseconds to wait=u32 1 ("等待时间（毫秒）")) -> ()  [unwired: 1 out]
    n7 = case shown="\"Calculate_and_check_tester_Parameter_after_Airwatts_Tune\"" w45 {
      selector: w45 -> [_ w64 w135 w181 w232 w350 w450 w548 w612 w653 w695 w740 w778 w825 w915 w992 w1066 w1122 w1188 w1253 w1298 w1340 w1404 w1450 w1497 w1554 w1607]
      tunnel: w46 -> [w51 w68 w142 w186 w242 w359 w459 w556 w625 w658 w708 w747 w784 w834 w924 w1000 w1079 w1131 w1198 w1263 w1305 w1350 w1414 w1457 w1507 w1564 w1616]
      tunnel: [w51 w68 w142 w186 w242 w359 w459 w556 w604 w658 w688 w747 w784 w834 w924 w1000 w1055 w1131 w1198 w1263 w1305 w1350 w1414 w1457 w1507 w1564 w1616] -> w44
      tunnel: w40 -> [w50 w67 _ w185 _ _ w458 w555 w629 w654 w712 _ w783 _ w923 w999 w1083 _ _ _ _ _ w1413 _ _ w1563 _]
      tunnel: [w50 w66 w141 w184 w241 w358 w457 w554 w626 w657 w709 w746 w782 w833 w922 w998 w1080 w1130 w1197 w1262 w1304 w1349 w1412 w1456 w1506 w1562 w1615] -> w39
      tunnel: [_ w61 w129 _ w223 w339 _ w535 w609 _ w687 w734 _ w818 _ _ w1062 w1119 w1182 w1247 w1295 w1334 w1399 w1445 w1491 w1549 TRUE] -> w24
      tunnel: w35 -> [w49 w58 w127 w179 w238 w355 w445 w546 w622 w652 w705 w731 w776 w830 w910 w989 w1076 w1127 w1194 w1259 w1293 w1346 w1410 w1443 w1503 w1560 w1613]
      tunnel: [w49 w58 w127 w179 w237 w354 w454 w552 w623 w652 w706 w731 w776 w829 w919 w996 w1077 w1126 w1193 w1258 w1293 w1345 w1409 w1443 w1502 w1559 w1612] -> w34
      tunnel: w31 -> [_ w65 w140 w183 w240 w357 w456 w553 w628 w656 w711 w745 w781 w832 w921 w997 w1082 w1129 w1196 w1261 w1303 w1348 w1411 w1455 w1505 w1561 w1614]
      tunnel: [_ w64 w135 w181 w232 w350 w450 w548 w612 w653 w695 w740 w778 w825 w915 w992 w1066 w1122 w1188 w1253 w1298 w1340 w1404 w1450 w1497 w1554 w1607] -> w30
      tunnel: w33 -> [_ w62 _ _ _ w332 _ _ _ _ _ _ _ _ _ _ _ _ _ _ w1288 _ _ _ _ _ _]
      tunnel: [_ "Max_Motor_On_with_power_mode" "MAX_Wait_for_X_sec_for_motor_speed_to_stabilise" w169 "Max_Get_and_check_DDM_Parameter" "Max_Get_and_check_tester_Parameter-A" "Max_Calculate_Tester_Parameter-B" w508 w611 w655 w686 "MAX_Wait_for_X_sec_for_motor_speed_to_stabilise_after_Airwatts_Tune" "Get_DDM_Parameter_after_Airwatts_Tune" "Get_tester_Parameter_after_Airwatts_Tune" "Calculate_and_check_tester_Parameter_after_Airwatts_Tune" w986 w1064 w1118 w1183 "Max_Stop_motor" w1287 "Max_Calculate_the_delta_pressure" w1375 "Max_Get_Cold_Bemf_in_mV" "Max_Calculate_and_Check_delta_BEMF" w1547 w1606] -> w32
      tunnel: [_ w54 w130 _ w224 w340 _ w508 w611 w655 w686 w735 _ w819 _ _ w1064 w1118 w1183 w1248 w1287 w1335 w1375 w1446 w1492 w1547 w1606] -> w29
      tunnel: w22 -> [w48 w57 w126 w176 w218 w337 w439 w525 w601 w645 w674 w730 w770 w800 w892 w972 w1045 w1115 w1178 w1246 w1292 w1333 w1383 w1442 w1490 w1544 w1597]
      tunnel: [w48 w56 w124 w175 w217 w335 w436 w524 w603 w645 w676 w729 w770 w799 w893 w971 w1054 w1112 w1172 w1243 w1289 w1331 w1392 w1439 w1487 w1543 w1593] -> w21
      tunnel: w20 -> [_ _ _ _ _ _ _ w512 w602 _ w675 _ _ _ _ _ w1046 w1103 w1163 _ _ _ w1385 w1430 _ w1534 w1584]
      frame "假", Default {
      }
      frame "MAX_Orifice_Size" {
        n8 = Unbundle By Name(w57) -> ("Config"=w60:string[][])
        n9 = call "Index_Config.vi"("Action"="MAX_POWER_MODE_Orifice_size", "config"=w60) -> ("data"=w55:string)  [unwired: 9 in]
        n10 = case shown="True" FALSE {
          tunnel: w62 -> [_ w87]
          tunnel: [_ w86] -> w61
          tunnel: [_ w85] -> w54
          tunnel: w55 -> [_ w84]
          frame False {
          }
          frame True {
            n11 = Unbundle By Name(w87) -> ("Motor.COM"=w78:refnum<visa-resource-name>)
            n12 = call "Position_Config.vi"("Step"=enum16{"Initial", "Write", "Read"}."Read") -> ("Position Config out"=w75:T11)  [unwired: 9 in, 1 out]
            n13 = case shown="\"12.7\", Default" w84 {
              tunnel: w75 -> [w89 w91 w93 w95]
              tunnel: [w88 w90 w92 w94] -> w74
              frame "12.7", Default {
                n14 = Unbundle By Name(w89) -> ("OrificeSize_12.7"=w88:i32)
              }
              frame "13" {
                n15 = Unbundle By Name(w91) -> ("OrificeSize_13"=w90:i32)
              }
              frame "30" {
                n16 = Unbundle By Name(w93) -> ("OrificeSize_30"=w92:i32)
              }
              frame "16" {
                n17 = Unbundle By Name(w95) -> ("OrificeSize_16"=w94:i32)
              }
            }
            n18 = call "IO.vi"("DO DATA"=bool[] [FALSE] ("Writel_IO"), "IO Name"=string[] ["Orifice_fixed_Cylinder"], "IO?"=enum16{"DI", "DO"}."DO") -> ("error out"=w70:errorcluster)  [unwired: 7 in, 1 out]
            n19 = To Long Integer(number=w74) -> (32bit integer=w80:i32)
            n20 = call "Time Delay"("error in (no error)"=w70) -> ("error out"=w69:errorcluster)  [unwired: 10 in]
            n21 = call "Pulse.vi"("Pulse"=w80) -> ("Pulse"=w81:string)  [unwired: 10 in]
            n22 = call "Motor Visa.vi"("错误输入（无错误）"=w69, "Command"=w81, "VISA资源名称"=w78) -> ("错误输出"=w82:errorcluster, "VISA资源名称输出"=w83:refnum<visa-resource-name>)  [unwired: 6 in, 1 out]
            n23 = call "ABS.vi"() -> ("绝对模式"=w79:string)  [unwired: 11 in]
            n24 = call "Motor Visa.vi"("错误输入（无错误）"=w82, "Command"=w79, "VISA资源名称"=w83) -> ("VISA资源名称输出"=w77:refnum<visa-resource-name>)  [unwired: 6 in, 2 out]
            n25 = while {
              tunnel: w77 -> [w121]
              tunnel: [w104] -> w86
              stop <- w111 stop-if-true
              n26 = call "Get Status.vi"() -> ("Command"=w122:string)  [unwired: 11 in]
              n27 = call "Get Alarm  Error Status.vi"() -> ("AlarmStatus"=w114:string, "ErrorStatus"=w115:string)  [unwired: 10 in]
              n28 = call "Motor Visa.vi"("Command"=w122, "VISA资源名称"=w121) -> ("读取缓冲区"=w120:string, "VISA资源名称输出"=w113:refnum<visa-resource-name>)  [unwired: 7 in, 1 out]
              n29 = Wait (ms)(milliseconds to wait=u32 50 ("等待时间（毫秒）")) -> ()  [unwired: 1 out]
              n30 = call "Motor Visa.vi"("Command"=w115, "VISA资源名称"=w113) -> ("读取缓冲区"=w117:string, "VISA资源名称输出"=w118:refnum<visa-resource-name>)  [unwired: 7 in, 1 out]
              n31 = call "Motor Visa.vi"("Command"=w114, "VISA资源名称"=w118) -> ("读取缓冲区"=w116:string)  [unwired: 7 in, 2 out]
              n32 = call "Exit.vi"("Step"=enum16{"Initial", "Write", "Read"}."Read" ("step")) -> ("Exit Out"=w107:bool)  [unwired: 9 in, 1 out]
              n33 = call "Stop.vi"("Step"=enum16{"Initial", "Write", "Read"}."Read") -> ("Stop Out"=w108:bool)  [unwired: 9 in, 1 out]
              n34 = call "Alarm and Error Result.vi"("Command"=w116) -> ("Alarm or Error"=w106:bool)  [unwired: 10 in]
              n35 = call "Alarm and Error Result.vi"("Command"=w117) -> ("Alarm or Error"=w105:bool)  [unwired: 10 in]
              n36 = call "Motion Down.vi"("Command"=w120) -> ("Motion Down"=w112:bool)  [unwired: 10 in]
              n37 = Compound Arithmetic op=OR(w107, w108, w106, w105, w112) -> (w111:bool)
              n38 = Or(x=w106, y=w105) -> (x .or. y?=w104:bool)
            }
            n39 = case shown="True" w86 {
              tunnel: [_ "Error" ("Message Name")] -> w85
              frame False {
                n40 = call "IO.vi"("DO DATA"=bool[] [TRUE] ("Writel_IO"), "IO Name"=string[] ["Orifice_fixed_Cylinder"], "IO?"=enum16{"DI", "DO"}."DO") -> ("error out"=w99:errorcluster)  [unwired: 7 in, 1 out]
                n41 = call "Time Delay2"("error in (no error)"=w99) -> ()  [unwired: 10 in, 1 out]
              }
              frame True {
                n42 = call "6-AlarmStatus.vi"("AlarmValue"=TRUE, "AlarmIndex"=AlarmIndex."Motor Error", "Step"=enum16{"Initial", "Write", "Read"}."Write") -> ()  [unwired: 7 in, 2 out]
              }
            }
          }
        }
        n43 = call "LogStatus.vi"("error in (no error)"=w67, "last message"=w65, "message"=w64) -> ("error  out"=w66:errorcluster)  [unwired: 8 in]
        n44 = Bundle By Name(cluster=w57, "MAX.Restriction Plate Diameter"=w55, "MAX_Status.Restriction Plate Diameter"="PASS") -> (w56:T1)
      }
      frame "Max_Motor_On_with_power_mode" {
        n45 = Unbundle By Name(w126) -> ("Table"=w134:string[][], "daemon reference"=w139:refnum<k5>, "Config"=w132:string[][])
        n46 = call "Select_Table_Vaule Enable_Disable.vi"("Action"=w135, "Table"=w134) -> ("Enable"=w136:bool)  [unwired: 8 in, 1 out]
        n47 = case shown="True" w136 {
          tunnel: w139 -> [w146 w164]
          tunnel: [TRUE w154] -> _
          tunnel: [w146 w158] -> w123
          tunnel: ["" ("response") w150] -> w128
          tunnel: w135 -> [_ w157]
          tunnel: w134 -> [_ w156]
          tunnel: w132 -> [_ w153]
          tunnel: "MAX_POWER_MODE_Drive_mode" -> [_ w152]
          tunnel: [_ w151] -> w125
          tunnel: [_ w150] -> _
          tunnel: [_ w149] -> _
          tunnel: [_ w148] -> _
          frame False {
          }
          frame True {
            w163 = "UIdisplay" ("Process (\"\" - local)")
            n48 = call "Index_Config.vi"("Action"=w152, "config"=w153) -> ("data"=w148:string)  [unwired: 9 in]
            n49 = call "drive_motor.vi"("Power Mode"=w148, "daemon reference in"=w164) -> ("error out"=w151:errorcluster, "response"=w150:string, "daemon reference out"=w158:refnum<k5>)  [unwired: 6 in, 1 out]
            n50 = call "Select_Table_Vaule.vi"("Vaule"=w150, "Action"=w157, "Table"=w156) -> ("Result"=w154:bool, "vaule"=w155:string[])  [unwired: 7 in]
            n51 = Append True/False String(1:w154, 2:"FAIL" ("真字符串"), 3:"PASS" ("真字符串")) -> (0:w149:string)  [unwired: 1 in]
            n52 = Build Array (concatenate)(w155, w150, w149) -> (w162:string[])
            n53 = Flatten To XML(anything=w162) -> (xml string=w161:string)
            n54 = call "AMC Send Local Message.vi"("Process (\"\" - local)"=w163, "Message Value"=w161, "Message Name"=w163) -> ()  [unwired: 7 in, 2 out]
          }
        }
        n55 = call <vilib>:"Space Constant.vi"() -> ("String"=w138:string)
        n56 = Concatenate Strings(w135, w138, w128) -> (w137:string)
        n57 = call "LogStatus.vi"("error in (no error)"=w125, "last message"=w140, "message"=w137) -> ("error  out"=w141:errorcluster)  [unwired: 8 in]
        n58 = Bundle By Name(cluster=w126, "daemon reference"=w123) -> (w124:T1)
        n59 = case shown="Error" w125 {
          tunnel: [_ TRUE] -> w129
          tunnel: [_ "Error"] -> w130
          frame No Error {
          }
          frame Error {
          }
        }
      }
      frame "MAX_Wait_for_X_sec_for_motor_speed_to_stabilise" {
        (unwired) "15" ("替换字符串(\"\")")
        # "来之Config"
        n60 = Unbundle By Name(w176) -> ("Config"=w178:string[][])
        n61 = call "Index_Config.vi"("Action"="MAX_POWER_MODE_Stabilisation_time" ("替换字符串(\"\")"), "config"=w178) -> ("data"=w174:string)  [unwired: 9 in]
        n62 = Get Date/Time In Seconds() -> (seconds since 1Jan1904=w167:timestamp)
        n63 = Search and Replace String(input string=w181, search string="X" ("搜索字符串"), replace string=w174) -> (result string=w182:string)  [unwired: 5 in, 3 out]
        n64 = call "LogStatus.vi"("error in (no error)"=w185, "last message"=w183, "message"=w182) -> ("error  out"=w184:errorcluster)  [unwired: 8 in]
        n65 = Fract/Exp String To Number(string=w174) -> (number=w166:dbl)  [unwired: 3 in, 1 out]
        n66 = while {
          tunnel: w167 -> [w193]
          tunnel: w166 -> [w190]
          tunnel: [w189] -> _
          stop <- w189 stop-if-true
          n67 = Get Date/Time In Seconds() -> (seconds since 1Jan1904=w194:timestamp)
          n68 = Subtract(x=w194, y=w193) -> (x-y=w192:dbl)
          n69 = call "6-AlarmStatus.vi"("Step"=enum16{"Initial", "Write", "Read"}."Read") -> ("AlarmValue Out"=w197:bool[])  [unwired: 9 in, 1 out]
          n70 = Greater Or Equal?(x=w192, y=w190) -> (x >= y?=w191:bool)
          n71 = call "Stop.vi"("Step"=enum16{"Initial", "Write", "Read"}."Read") -> ("Stop Out"=w195:bool)  [unwired: 9 in, 1 out]
          n72 = call "Exit.vi"("Step"=enum16{"Initial", "Write", "Read"}."Read" ("step")) -> ("Exit Out"=w199:bool)  [unwired: 9 in, 1 out]
          n73 = Or Array Elements(Boolean array=w197) -> (logical OR=w196:bool)
          n74 = Compound Arithmetic op=OR(w191, w195, w199, w196) -> (w189:bool)
          n75 = Wait (ms)(milliseconds to wait=u32 1 ("等待时间（毫秒）")) -> ()  [unwired: 1 out]
        }
        n76 = Bundle By Name(cluster=w176, "MAX.MAX - Stabilisation Time"=w174, "MAX_Status.MAX - Stabilisation Time"="PASS") -> (w175:T1)
        n77 = call "HD_Config.vi"("Step"=enum16{"Initial", "Write", "Read"}."Read") -> ("HD Config out"=w173:T5)  [unwired: 9 in, 1 out]
        n78 = Unbundle By Name(w173) -> ("GRR"=w171:bool)
        n79 = Select(t="Max_Get_and_check_DDM_Parameter", s=w171, f="Max_Collect_and_Calculate_Average_Delta_Tmag_LSI_and_FISF_data_every_one_sec_for_x_times") -> (s? t:f=w169:string)
      }
      frame "Max_Collect_and_Calculate_Average_Delta_Tmag_LSI_and_FISF_data_every_one_sec_for_x_times" {
        n80 = Unbundle By Name(w218) -> ("Table"=w231:string[][], "daemon reference"=w239:refnum<k5>, "Config"=w226:string[][])
        n81 = call "Select_Table_Vaule Enable_Disable.vi"("Action"=w232, "Table"=w231) -> ("Enable"=w233:bool)  [unwired: 8 in, 1 out]
        n82 = call "Index_Config.vi"("Action"="MAX_POWER_MODE_Average_Delta_Tmag_Time", "config"=w226) -> ("data"=w228:string)  [unwired: 9 in]
        n83 = Decimal String To Number(string=w228) -> (number=w225:i32)  [unwired: 2 in, 1 out]
        n84 = case shown="True" w233 {
          tunnel: w239 -> [w253 w275]
          tunnel: [w253 w274] -> w209
          tunnel: [w252 w259] -> w234
          tunnel: w232 -> [_ w261]
          tunnel: w231 -> [_ w276]
          tunnel: [_ w266] -> w229
          tunnel: w225 -> [_ w265]
          tunnel: [_ w264] -> w216
          tunnel: [_ w257] -> w211
          tunnel: [_ w256] -> w220
          tunnel: [w251 w255] -> w210
          tunnel: [w251 w254] -> w202
          frame False {
            w252 = "Skip" ("response")
            n85 = Initialize Array(w252, 6 ("维数大小")) -> (w251:string[])
          }
          frame True {
            n86 = Get Date/Time In Seconds() -> (seconds since 1Jan1904=w273:timestamp)
            n87 = while {
              shift-right: [w315] -> w274
              shift-left: w275 -> [w316]
              tunnel: w273 -> [w312]
              shift-right: [w308] -> w259
              shift-left: "" -> [w307]
              tunnel: [w305] -> w271 mode=indexing
              tunnel: [w304] -> w270 mode=indexing
              tunnel: [w303] -> w269 mode=indexing
              tunnel: [w302] -> w268 mode=indexing
              tunnel: [w301] -> w267 mode=indexing
              tunnel: w265 -> [w300]
              tunnel: [w298] -> w264
              stop <- w290 stop-if-true
              (unwired) enum16{"Initial", "Write", "Read"}."Read" ("Step")
              n88 = call "get_delta_tmag.vi"("daemon reference in"=w316) -> ("error out"=w299:errorcluster, "Tmag Data"=w306:T8, "response"=w311:string, "daemon reference out"=w315:refnum<k5>)  [unwired: 6 in, 1 out]
              n89 = call "Time Delay3"("error in (no error)"=w299) -> ("error out"=w298:errorcluster)  [unwired: 10 in]
              n90 = flat-sequence {
                tunnel: [w317] -> w313
                tunnel: w298 -> [_]
                frame #0 {
                  n91 = Get Date/Time In Seconds() -> (seconds since 1Jan1904=w317:timestamp)
                }
              }
              n92 = Unbundle By Name(w306) -> ("LSI Delta in degC"=w305:dbl, "FISF Delta in degc"=w304:dbl, "LSI Tmag in degC"=w303:dbl, "Fisf Tmag in degC"=w302:dbl, "IIR Tmag in degC"=w301:dbl)
              n93 = call "6-AlarmStatus.vi"("Step"=enum16{"Initial", "Write", "Read"}."Read") -> ("AlarmValue Out"=w294:bool[])  [unwired: 9 in, 1 out]
              n94 = Subtract(x=w313, y=w312) -> (x-y=w314:dbl)
              n95 = Concatenate Strings(w311, ";" ("字符串")) -> (w309:string)
              n96 = call "Stop.vi"() -> ("Stop Out"=w292:bool)  [unwired: 10 in, 1 out]
              n97 = call "Exit.vi"("Step"=enum16{"Initial", "Write", "Read"}."Read" ("step")) -> ("Exit Out"=w296:bool)  [unwired: 9 in, 1 out]
              n98 = Or Array Elements(Boolean array=w294) -> (logical OR=w293:bool)
              n99 = Greater Or Equal?(x=w314, y=w300) -> (x >= y?=w291:bool)
              n100 = Concatenate Strings(w307, w309) -> (w308:string)
              n101 = Compound Arithmetic op=OR(w291, w292, w296, w293) -> (w290:bool)
            }
            n102 = Build Array (concatenate)(w261, string[] ["Max_LSI_Delta_in_degC", "Max_FISF_Delta_in_degC", "Max_LSI_Tmag_in_degC", "Max_Fisf_Tmag_in_degC", "Max_IIR_Tmag_in_degC"]) -> (w260:string[])
            n103 = Build Array(w271, w270, w269, w268, w267) -> (w257:dbl[][])
            n104 = for {
              tunnel: w257 -> [w289] mode=indexing
              tunnel: [w288] -> w263 mode=indexing
              n105 = call-poly <vilib>:"Mean.vi"("X"=w289) -> ("mean"=w288:dbl)  [unwired: 1 out]
            }
            n106 = Array To Cluster(array=w263) -> (cluster=w266:T12)
            n107 = Number To Fractional String(number=w263) -> (F-format string=w255:string[])  [unwired: 3 in]
            n108 = Build Array (concatenate)(w259, w255) -> (w258:string[])
            n109 = for {
              tunnel: w276 -> [w282]
              tunnel: [w280] -> w256 mode=indexing
              tunnel: w258 -> [w279] mode=indexing
              tunnel: w260 -> [w278] mode=indexing
              tunnel: [w277] -> w254 mode=indexing
              w287 = "UIdisplay" ("Process (\"\" - local)")
              n110 = call "Select_Table_Vaule.vi"("Vaule"=w279, "Action"=w278, "Table"=w282) -> ("Result"=w280:bool, "vaule"=w281:string[])  [unwired: 7 in]
              n111 = Append True/False String(1:w280, 2:"FAIL" ("真字符串"), 3:"PASS" ("真字符串")) -> (0:w277:string)  [unwired: 1 in]
              n112 = Build Array (concatenate)(w281, w279, w277) -> (w286:string[])
              n113 = Flatten To XML(anything=w286) -> (xml string=w285:string)
              n114 = call "AMC Send Local Message.vi"("Process (\"\" - local)"=w287, "Message Value"=w285, "Message Name"=w287) -> ()  [unwired: 7 in, 2 out]
            }
          }
        }
        n115 = call <vilib>:"Space Constant.vi"() -> ("String"=w236:string)
        n116 = Concatenate Strings(w232, w236, w234) -> (w235:string)
        n117 = Transpose 2D Array(2D array=w211) -> (transposed array=w208:dbl[][])
        n118 = Index Array(array=w210, index=1 ("索引")) -> (element=w205:string)
        n119 = Index Array(array=w202, index=2 ("索引")) -> (element=w203:string)
        n120 = for {
          tunnel: w208 -> [w247] mode=indexing
          tunnel: [w243] -> w215 mode=indexing
          n121 = Array To Spreadsheet String(delimiter (Tab)=";", array=w247, 3:"" ("format string")) -> (spreadsheet string=w244:string)
          n122 = call <vilib>:"Trim Whitespace.vi"("string"=w244) -> ("trimmed string"=w243:string)  [unwired: 1 in]
        }
        n123 = Array To Spreadsheet String(delimiter (Tab)="|", array=w215, 3:"" ("format string")) -> (spreadsheet string=w214:string)
        n124 = Delete From Array(array=w220, length=1 ("长度"), index=0 ("索引")) -> (array with subset deleted=w219:bool[])  [unwired: 1 out]
        n125 = call <vilib>:"Trim Whitespace.vi"("string"=w214) -> ("trimmed string"=w207:string)  [unwired: 1 in]
        n126 = Bundle By Name(cluster=w218, "MAX_Status.Get Average Delta Tmag FISF"=w203, "MAX.Get Average Delta Tmag FISF"=w205, "MAX.Get Average Delta Tmag (LSIdelta_FISFdelta_LSItmag_FISFtmag_IIRtmag)"=w207, "daemon reference"=w209, "MAX_Status.Get Average Delta Tmag (LSIdelta_FISFdelta_LSItmag_FISFtmag_IIRtmag)"="PASS") -> (w217:T1)
        n127 = call "LogStatus.vi"("error in (no error)"=w216, "last message"=w240, "message"=w235) -> ("error  out"=w241:errorcluster)  [unwired: 8 in]
        n128 = Bundle By Name(cluster=w238, "MAX.Average_Tmag_Data_status"=w219, "MAX.Average_Tmag_Data"=w229, "MAX.Average_All_data"=w211) -> (w237:T3)
        n129 = case shown="Error" w216 {
          tunnel: [_ TRUE] -> w223
          tunnel: [_ "Error"] -> w224
          frame No Error {
          }
          frame Error {
          }
        }
      }
      frame "Max_Get_and_check_DDM_Parameter" {
        n130 = Unbundle By Name(w332) -> ("GRR"=w331:bool)
        n131 = Unbundle By Name(w337) -> ("Table"=w349:string[][], "daemon reference"=w356:refnum<k5>, "Config"=w347:string[][])
        n132 = case shown="False" w331 {
          tunnel: [T7[] ["voltage", "current", "power", "speed", "measured_power", "pressure"] ("Parameter") T7[] ["voltage", "current", "power", "speed", "measured_power", "pressure", "lsi_magnet_temp", "fisf_magnet_temp", "iir_magnet_temp"] ("Parameter")] -> w338
          frame False {
          }
          frame True {
          }
        }
        n133 = call "Select_Table_Vaule Enable_Disable.vi"("Action"=w350, "Table"=w349) -> ("Enable"=w348:bool)  [unwired: 8 in, 1 out]
        n134 = case shown="True" w348 {
          tunnel: w356 -> [w367 w394]
          tunnel: [w367 w393] -> w333
          tunnel: [w366 w385] -> w351
          tunnel: w350 -> [_ w390]
          tunnel: w349 -> [_ w395]
          tunnel: w347 -> [_ _]
          tunnel: [_ w379] -> w345
          tunnel: [_ w392] -> w344
          tunnel: [_ w383] -> w336
          tunnel: w338 -> [_ w378]
          tunnel: [w365 w373] -> w334
          tunnel: [w365 w369] -> w330
          tunnel: w331 -> [_ w368]
          frame False {
            w366 = "Skip" ("software string")
            n135 = Initialize Array(w366, 6 ("维数大小")) -> (w365:string[])
          }
          frame True {
            n136 = for {
              tunnel: [w403] -> w377 mode=indexing
              tunnel: [w402] -> w383
              tunnel: [w398] -> w380 mode=indexing
              tunnel: w378 -> [w400] mode=indexing
              shift-right: [w404] -> w393
              shift-left: w394 -> [w405]
              n137 = Build Array(w400) -> (w399:T7[])
              n138 = call "get_parameter.vi"("Parameter"=w399, "daemon reference in"=w405) -> ("error out"=w402:errorcluster, "response"=w403:string, "values"=w401:dbl[], "daemon reference out"=w404:refnum<k5>)  [unwired: 5 in, 1 out]
              n139 = Index Array(array=w401) -> (element=w398:dbl)  [unwired: 1 in]
            }
            n140 = case shown="True" w368 {
              tunnel: [string[] ["Max_DDM_Voltage", "Max_DDM_Current", "Max_DDM_Power", "Max_DDM_Speed", "Max_DDM_Measured_Power", "Max_DDM_Pressure"] string[] ["Max_DDM_Voltage", "Max_DDM_Current", "Max_DDM_Power", "Max_DDM_Speed", "Max_DDM_Measured_Power", "Max_DDM_Pressure", "Max_DDM_lsi_magnet_temp", "Max_DDM_fisf_magnet_temp", "Max_DDM_iir_magnet_temp"]] -> w384
              frame False {
              }
              frame True {
              }
            }
            n141 = Array To Spreadsheet String(delimiter (Tab)=",", array=w377, 3:"" ("format string")) -> (spreadsheet string=w376:string)
            n142 = in-place {
              w410 = 1000.0
              n143 = in-place-array #1(w380, 3, 5) -> (w409:dbl, w406:dbl)
              n144 = Divide(x=w409, y=w410) -> (x/y=w408:dbl)
              n145 = Divide(x=w406, y=w410) -> (x/y=w407:dbl)
              n146 = in-place-array #1(w408, w407) -> (w379:dbl[])  [unwired: 2 out]
            }
            n147 = Number To Fractional String(number=w379) -> (F-format string=w373:string[])  [unwired: 3 in]
            n148 = Interleave 1D Arrays(w384, w373) -> (w386:string[])
            n149 = Build Array (concatenate)(w376, w373) -> (w389:string[])
            n150 = Build Array (concatenate)(w390, w384) -> (w391:string[])
            n151 = Array To Spreadsheet String(delimiter (Tab)=";" ("分隔符(Tab)"), array=w386, 3:"" ("格式字符串")) -> (spreadsheet string=w385:string)
            n152 = for {
              tunnel: w395 -> [w417]
              tunnel: w389 -> [w415] mode=indexing
              tunnel: w391 -> [w414] mode=indexing
              tunnel: [w413] -> w392 mode=indexing
              tunnel: [w411] -> w370 mode=indexing
              w422 = "UIdisplay" ("Process (\"\" - local)")
              n153 = call "Select_Table_Vaule.vi"("Boolean"=TRUE, "Vaule"=w415, "Action"=w414, "Table"=w417) -> ("Result"=w413:bool, "vaule"=w416:string[])  [unwired: 6 in]
              n154 = Append True/False String(1:w413, 2:"FAIL" ("真字符串"), 3:"PASS" ("真字符串")) -> (0:w411:string)  [unwired: 1 in]
              n155 = Build Array (concatenate)(w416, w415, w411) -> (w421:string[])
              n156 = Flatten To XML(anything=w421) -> (xml string=w420:string)
              n157 = call "AMC Send Local Message.vi"("Process (\"\" - local)"=w422, "Message Value"=w420, "Message Name"=w422) -> ()  [unwired: 7 in, 2 out]
            }
            n158 = Delete From Array(array=w370, length=1 ("长度"), index=0 ("索引")) -> (array with subset deleted=w369:string[])  [unwired: 1 out]
          }
        }
        n159 = call <vilib>:"Space Constant.vi"() -> ("String"=w353:string)
        n160 = Concatenate Strings(w350, w353, w351) -> (w352:string)
        n161 = Index Array(array=w334) -> (element #1=w323:string, element #2=w322:string, element #3=w321:string, element #4=w319:string, element #5=w320:string, element #6=w318:string)  [unwired: 6 in]
        n162 = Index Array(array=w330) -> (element #1=w329:string, element #2=w328:string, element #3=w327:string, element #4=w325:string, element #5=w326:string, element #6=w324:string)  [unwired: 6 in]
        n163 = Bundle By Name(cluster=w337, "daemon reference"=w333, "MAX.MAX - DDM Parameter - Voltage"=w323, "MAX.MAX - DDM Parameter - Current"=w322, "MAX.MAX - DDM Parameter - Power"=w321, "MAX.MAX - DDM Parameter - Measured Power"=w320, "MAX.MAX - DDM Parameter - Speed"=w319, "MAX.MAX - DDM Parameter - Pressure"=w318, "MAX_Status.MAX - DDM Parameter - Voltage"=w329, "MAX_Status.MAX - DDM Parameter - Current"=w328, "MAX_Status.MAX - DDM Parameter - Power"=w327, "MAX_Status.MAX - DDM Parameter - Measured Power"=w326, "MAX_Status.MAX - DDM Parameter - Speed"=w325, "MAX_Status.MAX - DDM Parameter - Pressure"=w324, "MAX.MAX finetune - DDM Parameter - Voltage"=w323, "MAX.MAX finetune - DDM Parameter - Current"=w322, "MAX.MAX finetune - DDM Parameter - Power"=w321, "MAX.MAX finetune - DDM Parameter - Measured Power"=w320, "MAX.MAX finetune - DDM Parameter - Speed"=w319, "MAX.MAX finetune - DDM Parameter - Pressure"=w318) -> (w335:T1)
        n164 = call "LogStatus.vi"("error in (no error)"=w336, "last message"=w357, "message"=w352) -> ("error  out"=w358:errorcluster)  [unwired: 8 in]
        n165 = Delete From Array(array=w344, length=1 ("长度"), index=0 ("索引")) -> (array with subset deleted=w343:bool[])  [unwired: 1 out]
        n166 = Bundle By Name(cluster=w355, "MAX.DDM_Parameter"=w345, "MAX.DDM_Parameter_status"=w343) -> (w354:T3)
        n167 = case shown="Error" w336 {
          tunnel: [_ TRUE] -> w339
          tunnel: [_ "Error"] -> w340
          frame No Error {
          }
          frame Error {
          }
        }
      }
      frame "Max_Get_and_check_tester_Parameter-A" {
        n168 = Unbundle By Name(w439) -> ("Table"=w449:string[][], "daemon reference"=w455:refnum<k5>, "Config"=w447:string[][])
        n169 = call "Select_Table_Vaule Enable_Disable.vi"("Action"=w450, "Table"=w449) -> ("Enable"=w448:bool)  [unwired: 8 in, 1 out]
        n170 = case shown="True" w448 {
          tunnel: w455 -> [w463 w480]
          tunnel: [w463 w480] -> w437
          tunnel: [w462 w471] -> w451
          tunnel: w450 -> [_ w477]
          tunnel: w449 -> [_ w481]
          tunnel: w447 -> [_ _]
          tunnel: [_ w469] -> w446
          tunnel: [_ w479] -> w443
          tunnel: [w461 w466] -> w438
          tunnel: [w461 w464] -> w435
          frame False {
            w462 = "Skip" ("software string")
            n171 = Initialize Array(w462, 6 ("维数大小")) -> (w461:string[])
          }
          frame True {
            w470 = string[] ["Max_PM_Voltage", "Max_PM_Current", "Max_PM_Power", "Max_Ambient_Pressure", "Max_Ambient_Temperature", "Max_Ambient_humidity", "Max_Tester_Reference_Ambient_Pressure"]
            n172 = call "Power_Tunings_Tester_Parameter.vi"() -> ("Power_Tuning_Tester_Parameter"=w469:dbl[])  [unwired: 11 in]
            n173 = Number To Fractional String(number=w469) -> (F-format string=w466:string[])  [unwired: 3 in]
            n174 = Interleave 1D Arrays(w470, w466) -> (w472:string[])
            n175 = Array To Spreadsheet String(delimiter (Tab)=";" ("分隔符(Tab)"), array=w472, 3:"" ("格式字符串")) -> (spreadsheet string=w471:string)
            n176 = Build Array (concatenate)(w477, w470) -> (w478:string[])
            n177 = Build Array (concatenate)("", w466) -> (w476:string[])
            n178 = for {
              tunnel: w481 -> [w488]
              tunnel: w476 -> [w486] mode=indexing
              tunnel: w478 -> [w485] mode=indexing
              tunnel: [w484] -> w479 mode=indexing
              tunnel: [w482] -> w465 mode=indexing
              w493 = "UIdisplay" ("Process (\"\" - local)")
              n179 = call "Select_Table_Vaule.vi"("Boolean"=TRUE, "Vaule"=w486, "Action"=w485, "Table"=w488) -> ("Result"=w484:bool, "vaule"=w487:string[])  [unwired: 6 in]
              n180 = Append True/False String(1:w484, 2:"FAIL" ("真字符串"), 3:"PASS" ("真字符串")) -> (0:w482:string)  [unwired: 1 in]
              n181 = Build Array (concatenate)(w487, w486, w482) -> (w492:string[])
              n182 = Flatten To XML(anything=w492) -> (xml string=w491:string)
              n183 = call "AMC Send Local Message.vi"("Process (\"\" - local)"=w493, "Message Value"=w491, "Message Name"=w493) -> ()  [unwired: 7 in, 2 out]
            }
            n184 = Delete From Array(array=w465, length=1 ("长度"), index=0 ("索引")) -> (array with subset deleted=w464:string[])  [unwired: 1 out]
          }
        }
        n185 = call <vilib>:"Space Constant.vi"() -> ("String"=w453:string)
        n186 = Index Array(array=w438) -> (element #1=w428:string, element #2=w427:string, element #3=w426:string, element #4=w425:string, element #5=w424:string, element #6=w423:string)  [unwired: 6 in]
        n187 = Index Array(array=w435) -> (element #1=w434:string, element #2=w433:string, element #3=w432:string, element #4=w431:string, element #5=w430:string, element #6=w429:string)  [unwired: 6 in]
        n188 = Concatenate Strings(w450, w453, w451) -> (w452:string)
        n189 = Bundle By Name(cluster=w439, "daemon reference"=w437, "MAX.MAX - Tester Parameter - Voltage"=w428, "MAX.MAX - Tester Parameter - Current"=w427, "MAX.MAX - Tester Parameter - Power"=w426, "MAX.MAX - Tester Parameter - Ambient Pressure"=w425, "MAX.MAX - Tester Parameter - Ambient Temperature"=w424, "MAX.MAX - Tester Parameter - Ambient Humidity"=w423, "MAX_Status.MAX - Tester Parameter - Voltage"=w434, "MAX_Status.MAX - Tester Parameter - Current"=w433, "MAX_Status.MAX - Tester Parameter - Power"=w432, "MAX_Status.MAX - Tester Parameter - Ambient Pressure"=w431, "MAX_Status.MAX - Tester Parameter - Ambient Temperature"=w430, "MAX_Status.MAX - Tester Parameter - Ambient Humidity"=w429, "MAX.MAX finetune - Tester Parameter - Voltage"=w428, "MAX.MAX finetune - Tester Parameter - Current"=w427, "MAX.MAX finetune - Tester Parameter - Power"=w426, "MAX.MAX finetune - Tester Parameter - Ambient Pressure"=w425, "MAX.MAX finetune - Tester Parameter - Ambient Temperature"=w424, "MAX.MAX finetune - Tester Parameter - Ambient Humidity"=w423) -> (w436:T1)
        n190 = call "LogStatus.vi"("error in (no error)"=w458, "last message"=w456, "message"=w452) -> ("error  out"=w457:errorcluster)  [unwired: 8 in]
        n191 = Delete From Array(array=w443, length=1 ("长度"), index=0 ("索引")) -> (array with subset deleted=w442:bool[])  [unwired: 1 out]
        n192 = Bundle By Name(cluster=w445, "MAX.Get_Tester_Parameter"=w446, "MAX.Get_Tester_Parameter_status"=w442) -> (w454:T3)
      }
      frame "Max_Calculate_Tester_Parameter-B" {
        n193 = Unbundle By Name(w546) -> ("MAX.DDM_Parameter_status"=w531:bool[], "MAX.Get_Tester_Parameter_status"=w532:bool[], "MAX.DDM_Parameter"=w540:dbl[], "MAX.Get_Tester_Parameter"=w538:dbl[], "MAX.Average_Tmag_Data"=w534:T8)
        n194 = Unbundle By Name(w525) -> ("Table"=w528:string[][], "daemon reference"=w527:refnum<k5>, "Config"=w526:string[][])
        n195 = call "HD_Config.vi"("Step"=enum16{"Initial", "Write", "Read"}."Read") -> ("HD Config out"=w542:T5)  [unwired: 9 in, 1 out]
        n196 = Unbundle By Name(w542) -> ("FCO.COM"=w537:refnum<visa-resource-name>)
        n197 = call "Index_Config.vi"("Action"="MAX_POWER_MODE_Orifice_size", "config"=w526) -> ("data"=w539:string)  [unwired: 9 in]
        n198 = call "Select_Table_Vaule Enable_Disable.vi"("Action"=w548, "Table"=w528) -> ("Enable"=w547:bool)  [unwired: 8 in, 1 out]
        n199 = case shown="True" w547 {
          tunnel: w527 -> [w560 w588]
          tunnel: [w560 w588] -> w521
          tunnel: [w559 w580] -> w549
          tunnel: w548 -> [_ w586]
          tunnel: w528 -> [_ w589]
          tunnel: [_ w568] -> w523
          tunnel: w540 -> [_ w576]
          tunnel: w539 -> [_ w575]
          tunnel: w538 -> [_ w574]
          tunnel: w537 -> [_ w573]
          tunnel: [_ w571] -> w529
          tunnel: [w558 w564] -> w522
          tunnel: [w558 w562] -> w504
          tunnel: [_ w561] -> _
          frame False {
            w559 = "Skip" ("software string")
            n200 = Initialize Array(w559, 5 ("维数大小")) -> (w558:string[])
          }
          frame True {
            w579 = string[] ["Max_DDM_Pressure_corrected", "Max_DDM_Real_Power", "Max_Delta_V", "Max_Flow_rate", "Max_AW"]
            n201 = call "FCO_Read.vi"("VISA in"=w573) -> ("Pressure(Pa)"=w563:dbl)  [unwired: 7 in, 3 out]
            n202 = Fract/Exp String To Number(string=w575) -> (number=w578:dbl)  [unwired: 3 in, 1 out]
            n203 = call "AW_Calculate_Tester_Parameter.vi"("Tester Parameter"=w574, "DDM Parameter"=w576, "AW_Box_Pressure/Stag Total-Static Pressure rise"=w563, "Orifice_Plate_Diameter"=w578) -> ("Calculate Tester Parameter"=w577:dbl[])  [unwired: 7 in]
            n204 = Number To Fractional String(number=w563) -> (F-format string=w561:string)  [unwired: 3 in]
            n205 = Number To Fractional String(number=w577) -> (F-format string=w564:string[])  [unwired: 3 in]
            n206 = Interleave 1D Arrays(w579, w564) -> (w581:string[])
            n207 = Build Array (concatenate)("", w564) -> (w585:string[])
            n208 = Array To Spreadsheet String(delimiter (Tab)=";" ("分隔符(Tab)"), array=w581, 3:"" ("格式字符串")) -> (spreadsheet string=w580:string)
            n209 = Build Array (concatenate)(w586, w579) -> (w587:string[])
            n210 = for {
              tunnel: w589 -> [w595]
              tunnel: w585 -> [w593] mode=indexing
              tunnel: w587 -> [w592] mode=indexing
              tunnel: [w591] -> w572 mode=indexing
              tunnel: [w590] -> w565 mode=indexing
              w600 = "UIdisplay" ("Process (\"\" - local)")
              n211 = call "Select_Table_Vaule.vi"("Vaule"=w593, "Action"=w592, "Table"=w595) -> ("Result"=w591:bool, "vaule"=w594:string[])  [unwired: 7 in]
              n212 = Append True/False String(1:w591, 2:"FAIL" ("真字符串"), 3:"PASS" ("真字符串")) -> (0:w590:string)  [unwired: 1 in]
              n213 = Build Array (concatenate)(w594, w593, w590) -> (w599:string[])
              n214 = Flatten To XML(anything=w599) -> (xml string=w598:string)
              n215 = call "AMC Send Local Message.vi"("Process (\"\" - local)"=w600, "Message Value"=w598, "Message Name"=w600) -> ()  [unwired: 7 in, 2 out]
            }
            n216 = Build Array (concatenate)(w577, w563) -> (w568:dbl[])
            n217 = Delete From Array(array=w572, length=1, index=0) -> (array with subset deleted=w571:bool[])  [unwired: 1 out]
            n218 = Delete From Array(array=w565, length=1, index=0) -> (array with subset deleted=w562:string[])  [unwired: 1 out]
          }
        }
        n219 = Unbundle By Name(w512) -> ("MES bool"=w514:refnum<vi>)
        n220 = call "HD_Config.vi"("Step"=enum16{"Initial", "Write", "Read"}."Read") -> ("HD Config out"=w513:T5)  [unwired: 9 in, 1 out]
        n221 = Unbundle By Name(w513) -> ("GRR"=w505:bool, "Fail_resume_mode"=w515:bool)
        n222 = call <vilib>:"Space Constant.vi"() -> ("String"=w551:string)
        n223 = property class="Bool (严格)"(reference=w514) -> ("Value"=w516:bool)  [unwired: 1 in, 2 out]
        n224 = Not(x=w516) -> (.not. x?=w517:bool)
        n225 = Concatenate Strings(w548, w551, w549) -> (w550:string)
        n226 = Or(x=w515, y=w517) -> (x .or. y?=w519:bool)
        n227 = Build Array (concatenate)(w531, w532) -> (w530:bool[])
        n228 = And Array Elements(Boolean array=w530) -> (logical AND=w511:bool)
        n229 = Select(t=TRUE, s=w519, f=w511) -> (s? t:f=w506:bool)
        n230 = Index Array(array=w522) -> (element #1=w498:string, element #2=w497:string, element #3=w496:string, element #4=w495:string, element #5=w494:string)  [unwired: 5 in]
        n231 = Index Array(array=w504) -> (element #1=w503:string, element #2=w502:string, element #3=w501:string, element #4=w500:string, element #5=w499:string)  [unwired: 5 in]
        n232 = Bundle By Name(cluster=w525, "daemon reference"=w521, "MAX.MAX - Calculated Parameter - DDM Pressure Corrected"=w498, "MAX.MAX - Calculated Parameter - DDM Real Power"=w497, "MAX.MAX - Calculated Parameter - Delta V"=w496, "MAX.MAX - Calculated Parameter - Flowrate"=w495, "MAX.MAX - Calculated Parameter - Airwatt"=w494, "MAX_Status.MAX - Calculated Parameter - DDM Pressure Corrected"=w503, "MAX_Status.MAX - Calculated Parameter - DDM Real Power"=w502, "MAX_Status.MAX - Calculated Parameter - Delta V"=w501, "MAX_Status.MAX - Calculated Parameter - Flowrate"=w500, "MAX_Status.MAX - Calculated Parameter - Airwatt"=w499, "MAX.MAX finetune - Calculated Parameter - DDM Pressure Corrected"=w498, "MAX.MAX finetune - Calculated Parameter - DDM Real Power"=w497, "MAX.MAX finetune - Calculated Parameter - Delta V"=w496, "MAX.MAX finetune - Calculated Parameter - Flowrate"=w495, "MAX.MAX finetune - Calculated Parameter - Airwatt"=w494, "MAX.MAX tune - Calculated Parameter - Airwatt"=w494) -> (w524:T1)
        n233 = call "LogStatus.vi"("error in (no error)"=w555, "last message"=w553, "message"=w550) -> ("error  out"=w554:errorcluster)  [unwired: 8 in]
        n234 = Select(t=w534, s=w506, f=T8 {"LSI Delta in degC"=nan, "FISF Delta in degc"=nan, "LSI Tmag in degC"=nan, "Fisf Tmag in degC"=nan, "IIR Tmag in degC"=nan} ("Average_Tmag_Data")) -> (s? t:f=w536:T8)
        n235 = Select(t="BEMF_Finetune", s=w506, f="Finalization_NG_unit") -> (s? t:f=w509:string)
        n236 = Bundle By Name(cluster=w546, "MAX.Cal_Tester_Parameter"=w523, "MAX.Average_Tmag_Data"=w536, "MAX.Cal_Tester_Parameter_status"=w529) -> (w552:T3)
        n237 = Select(t="Max_Stop_motor", s=w505, f=w509) -> (s? t:f=w508:string)
        n238 = Select(t=w505, s=w505, f=w506) -> (s? t:f=w507:bool)
        n239 = Not(x=w507) -> (.not. x?=w535:bool)
      }
      frame "BEMF_Finetune" {
        w614 = "UIdisplay" ("Process (\"\" - local)")
        n240 = Unbundle By Name(w601) -> ("Table"=w613:string[][])
        n241 = call "Select_Table_Vaule Enable_Disable.vi"("Action"=w612, "Table"=w613) -> ("Enable"=w606:bool)  [unwired: 8 in, 1 out]
        n242 = call "LogStatus.vi"("error in (no error)"=w629, "last message"=w628, "message"=w612) -> ("error  out"=w627:errorcluster)  [unwired: 8 in]
        n243 = case shown="True" w606 {
          tunnel: w627 -> [w632 w644]
          tunnel: [w632 w643] -> w626
          tunnel: w625 -> [w634 w642]
          tunnel: [w634 w641] -> w624
          tunnel: [w633 w640] -> w623
          tunnel: ["Max_Check_AW" w639] -> w611
          tunnel: w622 -> [w633 w638]
          tunnel: w601 -> [w630 w637]
          tunnel: [w630 w636] -> w603
          tunnel: w602 -> [_ w635]
          frame False {
          }
          frame True {
            n244 = call "4.0.1_BEMF_Finetune.vi"("Data in"=w637, "error in (no error)"=w644, "AllControls In"=w635, 10:w638, "Message Queue out"=w642) -> ("error out"=w643:errorcluster, "Flow"=w639:string, "Data"=w640:T3, "Message Queue Out"=w641:T4, "Data out"=w636:T1)  [unwired: 2 in]
          }
        }
        n245 = Select(t="Enable" ("元素"), s=w606, f="Disable" ("元素")) -> (s? t:f=w605:string)
        n246 = call "Select_Table_Vaule.vi"("Vaule"=w605, "Action"=w612, "Table"=w613) -> ("Result"=w621:bool, "vaule"=w620:string[])  [unwired: 7 in]
        n247 = Flush Queue(queue=w624) -> (queue out=w604:T4)  [unwired: 1 in, 2 out]
        n248 = Append True/False String(1:w621, 2:"FAIL" ("真字符串"), 3:"PASS" ("真字符串")) -> (0:w619:string)  [unwired: 1 in]
        n249 = Build Array (concatenate)(w620, w605, w619) -> (w617:string[])
        n250 = Flatten To XML(anything=w617) -> (xml string=w618:string)
        n251 = call "AMC Send Local Message.vi"("Process (\"\" - local)"=w614, "Message Value"=w618, "Message Name"=w614) -> ()  [unwired: 7 in, 2 out]
        n252 = Equal?(x=w611, y="Error") -> (x = y?=w609:bool)
      }
      frame "Max_Check_AW" {
        n253 = flat-sequence {
          tunnel: w652 -> [w669]
          tunnel: [w662] -> w648
          tunnel: [w661] -> w647
          tunnel: [w659] -> w646
          tunnel: [w671] -> _
          tunnel: [w672] -> _
          tunnel: [w673] -> w649
          tunnel: w648 -> [w673]
          tunnel: w647 -> [w672]
          tunnel: w646 -> [w671]
          tunnel: [w670] -> _
          frame #0 {
            n254 = Unbundle By Name(w669) -> ("MAX.Cal_Tester_Parameter"=w665:dbl[], "MAX.Cal_Tester_Parameter_status"=w668:bool[])
            n255 = Index Array(array=w668, index=4) -> (element=w662:bool)
            n256 = Index Array(array=w665, index=4) -> (element=w660:dbl)
            n257 = Number To Fractional String(number=w660) -> (F-format string=w659:string)  [unwired: 3 in]
            n258 = Append True/False String(1:w662, 2:"FAIL" ("真字符串"), 3:"PASS" ("真字符串")) -> (0:w661:string)  [unwired: 1 in]
          }
          frame #1 {
            n259 = Get Date/Time In Seconds() -> (seconds since 1Jan1904=w670:timestamp)
          }
        }
        n260 = call "LogStatus.vi"("error in (no error)"=w654, "last message"=w656, "message"=w653) -> ("error  out"=w657:errorcluster)  [unwired: 8 in]
        n261 = Select(t="Max_check_derate_status", s=w649, f="Airwatts_Tune") -> (s? t:f=w655:string)
      }
      frame "Airwatts_Tune" {
        w697 = "UIdisplay" ("Process (\"\" - local)")
        n262 = Unbundle By Name(w675) -> ("MES bool"=w682:refnum<vi>)
        n263 = call "HD_Config.vi"("Step"=enum16{"Initial", "Write", "Read"}."Read") -> ("HD Config out"=w683:T5)  [unwired: 9 in, 1 out]
        n264 = Unbundle By Name(w683) -> ("Fail_resume_mode"=w681:bool)
        n265 = property class="Bool (严格)"(reference=w682) -> ("Value"=w680:bool)  [unwired: 1 in, 2 out]
        n266 = Not(x=w680) -> (.not. x?=w679:bool)
        n267 = Or(x=w681, y=w679) -> (x .or. y?=w677:bool)
        n268 = Unbundle By Name(w674) -> ("Table"=w696:string[][])
        n269 = call "Select_Table_Vaule Enable_Disable.vi"("Action"=w695, "Table"=w696) -> ("Enable"=w690:bool)  [unwired: 8 in, 1 out]
        n270 = call "LogStatus.vi"("error in (no error)"=w712, "last message"=w711, "message"=w695) -> ("error  out"=w710:errorcluster)  [unwired: 8 in]
        n271 = case shown="True" w690 {
          tunnel: w710 -> [w715 w727]
          tunnel: [w715 w726] -> w709
          tunnel: w708 -> [w717 w725]
          tunnel: [w717 w724] -> w707
          tunnel: [w716 w723] -> w706
          tunnel: ["Finalization_NG_unit" w722] -> w686
          tunnel: w705 -> [w716 w721]
          tunnel: w674 -> [w714 w719]
          tunnel: [w714 w718] -> w676
          tunnel: w677 -> [_ _]
          tunnel: w675 -> [_ w720]
          frame False {
          }
          frame True {
            n272 = call "4.0.2_Airwatts_Tune.vi"("Data in"=w719, "error in (no error)"=w727, "AllControls In"=w720, 10:w721, "Message Queue out"=w725) -> ("error out"=w726:errorcluster, "Flow"=w722:string, "Data"=w723:T3, "Message Queue Out"=w724:T4, "Data out"=w718:T1)  [unwired: 2 in]
          }
        }
        n273 = Select(t="Enable" ("元素"), s=w690, f="Disable" ("元素")) -> (s? t:f=w689:string)
        n274 = call "Select_Table_Vaule.vi"("Vaule"=w689, "Action"=w695, "Table"=w696) -> ("Result"=w704:bool, "vaule"=w703:string[])  [unwired: 7 in]
        n275 = Append True/False String(1:w704, 2:"FAIL" ("真字符串"), 3:"PASS" ("真字符串")) -> (0:w702:string)  [unwired: 1 in]
        n276 = Flush Queue(queue=w707) -> (queue out=w688:T4)  [unwired: 1 in, 2 out]
        n277 = Build Array (concatenate)(w703, w689, w702) -> (w700:string[])
        n278 = Flatten To XML(anything=w700) -> (xml string=w701:string)
        n279 = call "AMC Send Local Message.vi"("Process (\"\" - local)"=w697, "Message Value"=w701, "Message Name"=w697) -> ()  [unwired: 7 in, 2 out]
        n280 = Equal?(x=w686, y="Error") -> (x = y?=w693:bool)
        n281 = Equal?(x=w686, y="Finalization_NG_unit") -> (x = y?=w685:bool)
        n282 = Or(x=w693, y=w685) -> (x .or. y?=w687:bool)
      }
      frame "Motor_On_with_power_mode_after_Airwatts_Tune" {
        n283 = Unbundle By Name(w730) -> ("Table"=w739:string[][], "daemon reference"=w744:refnum<k5>, "Config"=w737:string[][])
        n284 = call "Select_Table_Vaule Enable_Disable.vi"("Action"=w740, "Table"=w739) -> ("Enable"=w741:bool)  [unwired: 8 in, 1 out]
        n285 = case shown="True" w741 {
          tunnel: w744 -> [w751 w769]
          tunnel: [TRUE w759] -> _
          tunnel: [w751 w763] -> w728
          tunnel: ["" ("response") w755] -> w732
          tunnel: w740 -> [_ w762]
          tunnel: w739 -> [_ w761]
          tunnel: w737 -> [_ w758]
          tunnel: "MAX_POWER_MODE_Drive_mode" -> [_ w757]
          tunnel: [_ w756] -> w733
          tunnel: [_ w755] -> _
          tunnel: [_ w754] -> _
          tunnel: [_ w753] -> _
          frame False {
          }
          frame True {
            (unwired) "B1" ("Power Mode")
            w768 = "UIdisplay" ("Process (\"\" - local)")
            n286 = call "Index_Config.vi"("Action"=w757, "config"=w758) -> ("data"=w753:string)  [unwired: 9 in]
            n287 = call "drive_motor.vi"("Power Mode"=w753, "daemon reference in"=w769) -> ("error out"=w756:errorcluster, "response"=w755:string, "daemon reference out"=w763:refnum<k5>)  [unwired: 6 in, 1 out]
            n288 = call "Select_Table_Vaule.vi"("Vaule"=w755, "Action"=w762, "Table"=w761) -> ("Result"=w759:bool, "vaule"=w760:string[])  [unwired: 7 in]
            n289 = Append True/False String(1:w759, 2:"FAIL" ("真字符串"), 3:"PASS" ("真字符串")) -> (0:w754:string)  [unwired: 1 in]
            n290 = Build Array (concatenate)(w760, w755, w754) -> (w767:string[])
            n291 = Flatten To XML(anything=w767) -> (xml string=w766:string)
            n292 = call "AMC Send Local Message.vi"("Process (\"\" - local)"=w768, "Message Value"=w766, "Message Name"=w768) -> ()  [unwired: 7 in, 2 out]
          }
        }
        n293 = call <vilib>:"Space Constant.vi"() -> ("String"=w743:string)
        n294 = Concatenate Strings(w740, w743, w732) -> (w742:string)
        n295 = Bundle By Name(cluster=w730, "daemon reference"=w728) -> (w729:T1)
        n296 = call "LogStatus.vi"("error in (no error)"=w733, "last message"=w745, "message"=w742) -> ("error  out"=w746:errorcluster)  [unwired: 8 in]
        n297 = case shown="Error" w733 {
          tunnel: [_ TRUE] -> w734
          tunnel: [_ "Error"] -> w735
          frame No Error {
          }
          frame Error {
          }
        }
      }
      frame "MAX_Wait_for_X_sec_for_motor_speed_to_stabilise_after_Airwatts_Tune" {
        (unwired) "15" ("替换字符串(\"\")")
        # "来之Config"
        n298 = Unbundle By Name(w770) -> ("Config"=w775:string[][])
        n299 = call "Index_Config.vi"("Action"="MAX_POWER_MODE_Stabilisation_Time_2(After_AW_Finetune) " ("替换字符串(\"\")"), "config"=w775) -> ("data"=w773:string)  [unwired: 9 in]
        n300 = Get Date/Time In Seconds() -> (seconds since 1Jan1904=w772:timestamp)
        n301 = Search and Replace String(input string=w778, search string="X" ("搜索字符串"), replace string=w773) -> (result string=w779:string)  [unwired: 5 in, 3 out]
        n302 = Fract/Exp String To Number(string=w773) -> (number=w771:dbl)  [unwired: 3 in, 1 out]
        n303 = while {
          tunnel: w772 -> [w791]
          tunnel: w771 -> [w788]
          tunnel: [w787] -> _
          stop <- w787 stop-if-true
          n304 = Get Date/Time In Seconds() -> (seconds since 1Jan1904=w792:timestamp)
          n305 = Subtract(x=w792, y=w791) -> (x-y=w790:dbl)
          n306 = call "6-AlarmStatus.vi"("Step"=enum16{"Initial", "Write", "Read"}."Read") -> ("AlarmValue Out"=w795:bool[])  [unwired: 9 in, 1 out]
          n307 = Greater Or Equal?(x=w790, y=w788) -> (x >= y?=w789:bool)
          n308 = call "Stop.vi"("Step"=enum16{"Initial", "Write", "Read"}."Read") -> ("Stop Out"=w793:bool)  [unwired: 9 in, 1 out]
          n309 = call "Exit.vi"("Step"=enum16{"Initial", "Write", "Read"}."Read" ("step")) -> ("Exit Out"=w797:bool)  [unwired: 9 in, 1 out]
          n310 = Or Array Elements(Boolean array=w795) -> (logical OR=w794:bool)
          n311 = Compound Arithmetic op=OR(w789, w793, w797, w794) -> (w787:bool)
          n312 = Wait (ms)(milliseconds to wait=u32 1 ("等待时间（毫秒）")) -> ()  [unwired: 1 out]
        }
        n313 = call "LogStatus.vi"("error in (no error)"=w783, "last message"=w781, "message"=w779) -> ("error  out"=w782:errorcluster)  [unwired: 8 in]
      }
      frame "Get_DDM_Parameter_after_Airwatts_Tune" {
        n314 = Unbundle By Name(w800) -> ("Table"=w824:string[][], "daemon reference"=w831:refnum<k5>, "Config"=w822:string[][])
        n315 = call "Select_Table_Vaule Enable_Disable.vi"("Action"=w825, "Table"=w824) -> ("Enable"=w823:bool)  [unwired: 8 in, 1 out]
        n316 = case shown="False" w823 {
          tunnel: w831 -> [w840 w865]
          tunnel: [w840 w864] -> w801
          tunnel: [w839 w857] -> w826
          tunnel: w825 -> [_ w862]
          tunnel: w824 -> [_ w866]
          tunnel: w822 -> [_ _]
          tunnel: [_ w851] -> w820
          tunnel: [_ w855] -> w816
          tunnel: T7[] ["voltage", "current", "power", "speed", "measured_power", "pressure", "lsi_magnet_temp", "fisf_magnet_temp", "iir_magnet_temp"] ("Parameter") -> [_ w850]
          tunnel: [w838 w845] -> w802
          tunnel: [w838 w841] -> w803
          frame False {
            w839 = "Skip" ("software string")
            n317 = Initialize Array(w839, 6 ("维数大小")) -> (w838:string[])
          }
          frame True {
            w856 = string[] ["DDM_voltage_after_Airwatts_Tune", "DDM_current_after_Airwatts_Tune", "DDM_power_after_Airwatts_Tune", "DDM_speed_after_Airwatts_Tune", "DDM_measured_power_after_Airwatts_Tune", "DDM_pressure_after_Airwatts_Tune", "DDM_lsi_magnet_temp_after_Airwatts_Tune", "DDM_fisf_magnet_temp_after_Airwatts_Tune", "DDM_iir_magnet_temp_after_Airwatts_Tune"]
            n318 = for {
              tunnel: [w872] -> w849 mode=indexing
              tunnel: [w871] -> w855
              tunnel: [w867] -> w852 mode=indexing
              tunnel: w850 -> [w869] mode=indexing
              shift-right: [w873] -> w864
              shift-left: w865 -> [w874]
              n319 = Build Array(w869) -> (w868:T7[])
              n320 = call "get_parameter.vi"("Parameter"=w868, "daemon reference in"=w874) -> ("error out"=w871:errorcluster, "response"=w872:string, "values"=w870:dbl[], "daemon reference out"=w873:refnum<k5>)  [unwired: 5 in, 1 out]
              n321 = Index Array(array=w870) -> (element=w867:dbl)  [unwired: 1 in]
            }
            n322 = in-place {
              w879 = 1000.0
              n323 = in-place-array #2(w852, 3, 5) -> (w878:dbl, w875:dbl)
              n324 = Divide(x=w878, y=w879) -> (x/y=w877:dbl)
              n325 = Divide(x=w875, y=w879) -> (x/y=w876:dbl)
              n326 = in-place-array #2(w877, w876) -> (w851:dbl[])  [unwired: 2 out]
            }
            n327 = Array To Spreadsheet String(delimiter (Tab)=",", array=w849, 3:"" ("format string")) -> (spreadsheet string=w848:string)
            n328 = Number To Fractional String(number=w851) -> (F-format string=w845:string[])  [unwired: 3 in]
            n329 = Interleave 1D Arrays(w856, w845) -> (w858:string[])
            n330 = Build Array (concatenate)(w848, w845) -> (w861:string[])
            n331 = Array To Spreadsheet String(delimiter (Tab)=";" ("分隔符(Tab)"), array=w858, 3:"" ("格式字符串")) -> (spreadsheet string=w857:string)
            n332 = Build Array (concatenate)(w862, w856) -> (w863:string[])
            n333 = for {
              tunnel: w866 -> [w886]
              tunnel: w861 -> [w884] mode=indexing
              tunnel: w863 -> [w883] mode=indexing
              tunnel: [w880] -> w842 mode=indexing
              w891 = "UIdisplay" ("Process (\"\" - local)")
              n334 = call "Select_Table_Vaule.vi"("Boolean"=TRUE, "Vaule"=w884, "Action"=w883, "Table"=w886) -> ("Result"=w882:bool, "vaule"=w885:string[])  [unwired: 6 in]
              n335 = Append True/False String(1:w882, 2:"FAIL" ("真字符串"), 3:"PASS" ("真字符串")) -> (0:w880:string)  [unwired: 1 in]
              n336 = Build Array (concatenate)(w885, w884, w880) -> (w890:string[])
              n337 = Flatten To XML(anything=w890) -> (xml string=w889:string)
              n338 = call "AMC Send Local Message.vi"("Process (\"\" - local)"=w891, "Message Value"=w889, "Message Name"=w891) -> ()  [unwired: 7 in, 2 out]
            }
            n339 = Delete From Array(array=w842, length=1, index=0) -> (array with subset deleted=w841:string[])  [unwired: 1 out]
          }
        }
        n340 = call <vilib>:"Space Constant.vi"() -> ("String"=w828:string)
        n341 = Concatenate Strings(w825, w828, w826) -> (w827:string)
        n342 = Index Array(array=w802) -> (element #1=w815:string, element #2=w814:string, element #3=w813:string, element #4=w812:string, element #5=w811:string, element #6=w810:string)  [unwired: 6 in]
        n343 = Index Array(array=w803) -> (element #1=w809:string, element #2=w808:string, element #3=w807:string, element #4=w805:string, element #5=w806:string, element #6=w804:string)  [unwired: 6 in]
        n344 = Bundle By Name(cluster=w800, "daemon reference"=w801, "MAX.MAX finetune - DDM Parameter - Voltage"=w815, "MAX.MAX finetune - DDM Parameter - Current"=w814, "MAX.MAX finetune - DDM Parameter - Power"=w813, "MAX.MAX finetune - DDM Parameter - Measured Power"=w811, "MAX.MAX finetune - DDM Parameter - Speed"=w812, "MAX.MAX finetune - DDM Parameter - Pressure"=w810, "MAX_Status.MAX finetune - DDM Parameter - Voltage"=w809, "MAX_Status.MAX finetune - DDM Parameter - Current"=w808, "MAX_Status.MAX finetune - DDM Parameter - Power"=w807, "MAX_Status.MAX finetune - DDM Parameter - Measured Power"=w806, "MAX_Status.MAX finetune - DDM Parameter - Speed"=w805, "MAX_Status.MAX finetune - DDM Parameter - Pressure"=w804) -> (w799:T1)
        n345 = call "LogStatus.vi"("error in (no error)"=w816, "last message"=w832, "message"=w827) -> ("error  out"=w833:errorcluster)  [unwired: 8 in]
        n346 = Bundle By Name(cluster=w830, "MAX.DDM_Parameter_after_Airwatts_Tune"=w820) -> (w829:T3)
        n347 = case shown="Error" w816 {
          tunnel: [_ TRUE] -> w818
          tunnel: [_ "Error"] -> w819
          frame No Error {
          }
          frame Error {
          }
        }
      }
      frame "Get_tester_Parameter_after_Airwatts_Tune" {
        n348 = Unbundle By Name(w892) -> ("Table"=w914:string[][], "daemon reference"=w920:refnum<k5>, "Config"=w912:string[][])
        n349 = call "Select_Table_Vaule Enable_Disable.vi"("Action"=w915, "Table"=w914) -> ("Enable"=w913:bool)  [unwired: 8 in, 1 out]
        n350 = case shown="False" w913 {
          tunnel: w920 -> [w928 w944]
          tunnel: [w928 w944] -> w894
          tunnel: [w927 w936] -> w916
          tunnel: w915 -> [_ w942]
          tunnel: w914 -> [_ w945]
          tunnel: w912 -> [_ _]
          tunnel: [_ w934] -> w911
          tunnel: [w926 w930] -> w895
          tunnel: [w926 w929] -> w896
          frame False {
            w927 = "Skip" ("software string")
            n351 = Initialize Array(w927, 6 ("维数大小")) -> (w926:string[])
          }
          frame True {
            w935 = string[] ["Tester_Voltage_after_Airwatts_Tune", "Tester_Current_after_Airwatts_Tune", "Tester_Power_after_Airwatts_Tune", "Tester_Ambient_Pressure_after_Airwatts_Tune", "Tester_Ambient_Temperature_after_Airwatts_Tune", "Tester_Ambient_humidity_after_Airwatts_Tune", "Tester_Reference_Ambient_Pressure_after_Airwatts_Tune"]
            n352 = call "Power_Tunings_Tester_Parameter.vi"() -> ("Power_Tuning_Tester_Parameter"=w934:dbl[])  [unwired: 11 in]
            n353 = Number To Fractional String(number=w934) -> (F-format string=w930:string[])  [unwired: 3 in]
            n354 = Interleave 1D Arrays(w935, w930) -> (w937:string[])
            n355 = Array To Spreadsheet String(delimiter (Tab)=";" ("分隔符(Tab)"), array=w937, 3:"" ("格式字符串")) -> (spreadsheet string=w936:string)
            n356 = Build Array (concatenate)(w942, w935) -> (w943:string[])
            n357 = Build Array (concatenate)("", w930) -> (w941:string[])
            n358 = for {
              tunnel: w945 -> [w952]
              tunnel: w941 -> [w950] mode=indexing
              tunnel: w943 -> [w949] mode=indexing
              tunnel: [w946] -> w931 mode=indexing
              w957 = "UIdisplay" ("Process (\"\" - local)")
              n359 = call "Select_Table_Vaule.vi"("Boolean"=TRUE, "Vaule"=w950, "Action"=w949, "Table"=w952) -> ("Result"=w948:bool, "vaule"=w951:string[])  [unwired: 6 in]
              n360 = Append True/False String(1:w948, 2:"FAIL" ("真字符串"), 3:"PASS" ("真字符串")) -> (0:w946:string)  [unwired: 1 in]
              n361 = Build Array (concatenate)(w951, w950, w946) -> (w956:string[])
              n362 = Flatten To XML(anything=w956) -> (xml string=w955:string)
              n363 = call "AMC Send Local Message.vi"("Process (\"\" - local)"=w957, "Message Value"=w955, "Message Name"=w957) -> ()  [unwired: 7 in, 2 out]
            }
            n364 = Delete From Array(array=w931, length=1, index=0) -> (array with subset deleted=w929:string[])  [unwired: 1 out]
          }
        }
        n365 = call <vilib>:"Space Constant.vi"() -> ("String"=w918:string)
        n366 = Concatenate Strings(w915, w918, w916) -> (w917:string)
        n367 = Index Array(array=w896) -> (element #1=w902:string, element #2=w901:string, element #3=w900:string, element #4=w899:string, element #5=w898:string, element #6=w897:string)  [unwired: 6 in]
        n368 = Index Array(array=w895) -> (element #1=w908:string, element #2=w907:string, element #3=w906:string, element #4=w905:string, element #5=w904:string, element #6=w903:string)  [unwired: 6 in]
        n369 = Bundle By Name(cluster=w892, "daemon reference"=w894, "MAX.MAX finetune - Tester Parameter - Voltage"=w908, "MAX.MAX finetune - Tester Parameter - Current"=w907, "MAX.MAX finetune - Tester Parameter - Power"=w906, "MAX.MAX finetune - Tester Parameter - Ambient Pressure"=w905, "MAX.MAX finetune - Tester Parameter - Ambient Temperature"=w904, "MAX.MAX finetune - Tester Parameter - Ambient Humidity"=w903, "MAX_Status.MAX finetune - Tester Parameter - Voltage"=w902, "MAX_Status.MAX finetune - Tester Parameter - Current"=w901, "MAX_Status.MAX finetune - Tester Parameter - Power"=w900, "MAX_Status.MAX finetune - Tester Parameter - Ambient Pressure"=w899, "MAX_Status.MAX finetune - Tester Parameter - Ambient Temperature"=w898, "MAX_Status.MAX finetune - Tester Parameter - Ambient Humidity"=w897) -> (w893:T1)
        n370 = call "LogStatus.vi"("error in (no error)"=w923, "last message"=w921, "message"=w917) -> ("error  out"=w922:errorcluster)  [unwired: 8 in]
        n371 = Bundle By Name(cluster=w910, "MAX.Get_Tester_Parameter_after_Airwatts_Tune"=w911) -> (w919:T3)
      }
      frame "Calculate_and_check_tester_Parameter_after_Airwatts_Tune" {
        n372 = Unbundle By Name(w989) -> ("MAX.DDM_Parameter_after_Airwatts_Tune"=w981:dbl[], "MAX.Get_Tester_Parameter_after_Airwatts_Tune"=w980:dbl[])
        n373 = Unbundle By Name(w972) -> ("Table"=w975:string[][], "daemon reference"=w974:refnum<k5>, "Config"=w973:string[][])
        n374 = call "HD_Config.vi"("Step"=enum16{"Initial", "Write", "Read"}."Read") -> ("HD Config out"=w983:T5)  [unwired: 9 in, 1 out]
        n375 = Unbundle By Name(w983) -> ("FCO.COM"=w979:refnum<visa-resource-name>)
        n376 = call "Index_Config.vi"("Action"="MAX_POWER_MODE_Orifice_size", "config"=w973) -> ("data"=w978:string)  [unwired: 9 in]
        n377 = call "Select_Table_Vaule Enable_Disable.vi"("Action"=w992, "Table"=w975) -> ("Enable"=w991:bool)  [unwired: 8 in, 1 out]
        n378 = case shown="True" w991 {
          tunnel: w974 -> [w1004 w1032]
          tunnel: [w1004 w1032] -> w969
          tunnel: [w1003 w1023] -> w993
          tunnel: w992 -> [_ w1030]
          tunnel: w975 -> [_ w1033]
          tunnel: [_ w1012] -> w990
          tunnel: [_ w1015] -> w985
          tunnel: w981 -> [_ w1020]
          tunnel: w980 -> [_ w1019]
          tunnel: w979 -> [_ w1018]
          tunnel: w978 -> [_ w1017]
          tunnel: [w1002 w1011] -> w970
          tunnel: [w1002 w1007] -> w968
          tunnel: [_ w1005] -> _
          frame False {
            w1003 = "Skip" ("software string")
            n379 = Initialize Array(w1003, 5 ("维数大小")) -> (w1002:string[])
          }
          frame True {
            w1024 = string[] ["DDM_Pressure_corrected_after_Airwatts_Tune", "DDM_Real_Power_after_Airwatts_Tune", "Delta_V_after_Airwatts_Tune", "Flow_rate_after_Airwatts_Tune", "AW_after_Airwatts_Tune"]
            n380 = call "FCO_Read.vi"("VISA in"=w1018) -> ("Pressure(Pa)"=w1006:dbl)  [unwired: 7 in, 3 out]
            n381 = Fract/Exp String To Number(string=w1017) -> (number=w1022:dbl)  [unwired: 3 in, 1 out]
            n382 = call "AW_Calculate_Tester_Parameter.vi"("Tester Parameter"=w1019, "DDM Parameter"=w1020, "AW_Box_Pressure/Stag Total-Static Pressure rise"=w1006, "Orifice_Plate_Diameter"=w1022) -> ("Calculate Tester Parameter"=w1021:dbl[])  [unwired: 7 in]
            n383 = Number To Fractional String(number=w1006) -> (F-format string=w1005:string)  [unwired: 3 in]
            n384 = Number To Fractional String(number=w1021) -> (F-format string=w1011:string[])  [unwired: 3 in]
            n385 = Interleave 1D Arrays(w1024, w1011) -> (w1025:string[])
            n386 = Build Array (concatenate)(w1030, w1024) -> (w1031:string[])
            n387 = Array To Spreadsheet String(delimiter (Tab)=";" ("分隔符(Tab)"), array=w1025, 3:"" ("格式字符串")) -> (spreadsheet string=w1023:string)
            n388 = Build Array (concatenate)("", w1011) -> (w1029:string[])
            n389 = for {
              tunnel: w1033 -> [w1039]
              tunnel: w1029 -> [w1037] mode=indexing
              tunnel: w1031 -> [w1036] mode=indexing
              tunnel: [w1035] -> w1016 mode=indexing
              tunnel: [w1034] -> w1008 mode=indexing
              w1044 = "UIdisplay" ("Process (\"\" - local)")
              n390 = call "Select_Table_Vaule.vi"("Vaule"=w1037, "Action"=w1036, "Table"=w1039) -> ("Result"=w1035:bool, "vaule"=w1038:string[])  [unwired: 7 in]
              n391 = Append True/False String(1:w1035, 2:"FAIL" ("真字符串"), 3:"PASS" ("真字符串")) -> (0:w1034:string)  [unwired: 1 in]
              n392 = Build Array (concatenate)(w1038, w1037, w1034) -> (w1043:string[])
              n393 = Flatten To XML(anything=w1043) -> (xml string=w1042:string)
              n394 = call "AMC Send Local Message.vi"("Process (\"\" - local)"=w1044, "Message Value"=w1042, "Message Name"=w1044) -> ()  [unwired: 7 in, 2 out]
            }
            n395 = Build Array (concatenate)(w1021, w1006) -> (w1012:dbl[])
            n396 = Delete From Array(array=w1008, length=1, index=0) -> (array with subset deleted=w1007:string[])  [unwired: 1 out]
            n397 = Delete From Array(array=w1016, length=1, index=0) -> (array with subset deleted=w1015:bool[])  [unwired: 1 out]
          }
        }
        n398 = call <vilib>:"Space Constant.vi"() -> ("String"=w995:string)
        n399 = Concatenate Strings(w992, w995, w993) -> (w994:string)
        n400 = Index Array(array=w970) -> (element #1=w967:string, element #2=w966:string, element #3=w965:string, element #4=w964:string, element #5=w963:string)  [unwired: 5 in]
        n401 = Index Array(array=w968) -> (element #1=w962:string, element #2=w961:string, element #3=w960:string, element #4=w959:string, element #5=w958:string)  [unwired: 5 in]
        n402 = Index Array(array=w985, index=4) -> (element=w977:bool)
        n403 = Bundle By Name(cluster=w972, "daemon reference"=w969, "MAX.MAX tune - Calculated Parameter - Airwatt"=w963, "MAX_Status.MAX tune - Calculated Parameter - Airwatt"=w958, "MAX.MAX finetune - Calculated Parameter - DDM Pressure Corrected"=w967, "MAX.MAX finetune - Calculated Parameter - DDM Real Power"=w966, "MAX.MAX finetune - Calculated Parameter - Delta V"=w965, "MAX.MAX finetune - Calculated Parameter - Flowrate"=w964, "MAX.MAX finetune - Calculated Parameter - Airwatt"=w963, "MAX_Status.MAX finetune - Calculated Parameter - DDM Pressure Corrected"=w962, "MAX_Status.MAX finetune - Calculated Parameter - DDM Real Power"=w961, "MAX_Status.MAX finetune - Calculated Parameter - Delta V"=w960, "MAX_Status.MAX finetune - Calculated Parameter - Flowrate"=w959, "MAX_Status.MAX finetune - Calculated Parameter - Airwatt"=w958) -> (w971:T1)
        n404 = call "LogStatus.vi"("error in (no error)"=w999, "last message"=w997, "message"=w994) -> ("error  out"=w998:errorcluster)  [unwired: 8 in]
        n405 = Bundle By Name(cluster=w989, "MAX.Cal_Tester_Parameter_after_Airwatts_Tune"=w990, "MAX.Cal_Tester_Parameter_status_after_Airwatts_Tune"=w985) -> (w996:T3)
        n406 = Select(t="Max_check_derate_status", s=w977, f="Airwatts_Finetune") -> (s? t:f=w986:string)
      }
      frame "Airwatts_Finetune" {
        w1068 = "UIdisplay" ("Process (\"\" - local)")
        n407 = Unbundle By Name(w1046) -> ("MES bool"=w1052:refnum<vi>)
        n408 = call "HD_Config.vi"("Step"=enum16{"Initial", "Write", "Read"}."Read") -> ("HD Config out"=w1053:T5)  [unwired: 9 in, 1 out]
        n409 = Unbundle By Name(w1053) -> ("Fail_resume_mode"=w1051:bool)
        n410 = property class="Bool (严格)"(reference=w1052) -> ("Value"=w1050:bool)  [unwired: 1 in, 2 out]
        n411 = Not(x=w1050) -> (.not. x?=w1049:bool)
        n412 = Or(x=w1051, y=w1049) -> (x .or. y?=w1047:bool)
        n413 = Unbundle By Name(w1045) -> ("Table"=w1067:string[][])
        n414 = call "Select_Table_Vaule Enable_Disable.vi"("Action"=w1066, "Table"=w1067) -> ("Enable"=w1057:bool)  [unwired: 8 in, 1 out]
        n415 = call "LogStatus.vi"("error in (no error)"=w1083, "last message"=w1082, "message"=w1066) -> ("error  out"=w1081:errorcluster)  [unwired: 8 in]
        n416 = case shown="True" w1057 {
          tunnel: w1081 -> [w1086 w1098]
          tunnel: [w1086 w1097] -> w1080
          tunnel: w1079 -> [w1088 w1096]
          tunnel: [w1088 w1095] -> w1078
          tunnel: [w1087 w1094] -> w1077
          tunnel: ["Finalization_NG_unit" w1093] -> w1064
          tunnel: w1076 -> [w1087 w1092]
          tunnel: w1045 -> [w1084 w1090]
          tunnel: [w1084 w1091] -> w1054
          tunnel: w1047 -> [_ _]
          tunnel: w1046 -> [_ w1089]
          frame False {
          }
          frame True {
            n417 = call "4.0.3_Airwatts_Finetune.vi"("Data in"=w1090, "error in (no error)"=w1098, "AllControls In"=w1089, 10:w1092, "Message Queue out"=w1096) -> ("error out"=w1097:errorcluster, "Flow"=w1093:string, "Data"=w1094:T3, "Message Queue Out"=w1095:T4, "Data out"=w1091:T1)  [unwired: 2 in]
          }
        }
        n418 = Select(t="Enable" ("元素"), s=w1057, f="Disable" ("元素")) -> (s? t:f=w1056:string)
        n419 = call "Select_Table_Vaule.vi"("Vaule"=w1056, "Action"=w1066, "Table"=w1067) -> ("Result"=w1075:bool, "vaule"=w1074:string[])  [unwired: 7 in]
        n420 = Append True/False String(1:w1075, 2:"FAIL" ("真字符串"), 3:"PASS" ("真字符串")) -> (0:w1073:string)  [unwired: 1 in]
        n421 = Build Array (concatenate)(w1074, w1056, w1073) -> (w1071:string[])
        n422 = Flush Queue(queue=w1078) -> (queue out=w1055:T4)  [unwired: 1 in, 2 out]
        n423 = Flatten To XML(anything=w1071) -> (xml string=w1072:string)
        n424 = call "AMC Send Local Message.vi"("Process (\"\" - local)"=w1068, "Message Value"=w1072, "Message Name"=w1068) -> ()  [unwired: 7 in, 2 out]
        n425 = Equal?(x=w1064, y="Finalization_NG_unit") -> (x = y?=w1061:bool)
        n426 = Equal?(x=w1064, y="Error") -> (x = y?=w1060:bool)
        n427 = Or(x=w1061, y=w1060) -> (x .or. y?=w1062:bool)
      }
      frame "Max_check_derate_status" {
        n428 = Unbundle By Name(w1115) -> ("Table"=w1121:string[][], "daemon reference"=w1128:refnum<k5>, "Config"=w1120:string[][])
        n429 = Unbundle By Name(w1103) -> ("MES bool"=w1105:refnum<vi>)
        n430 = call "HD_Config.vi"("Step"=enum16{"Initial", "Write", "Read"}."Read") -> ("HD Config out"=w1104:T5)  [unwired: 9 in, 1 out]
        n431 = call "Select_Table_Vaule Enable_Disable.vi"("Action"=w1122, "Table"=w1121) -> ("Enable"=w1123:bool)  [unwired: 8 in, 1 out]
        n432 = case shown="False" w1123 {
          tunnel: w1128 -> [w1139 w1156]
          tunnel: [TRUE w1143] -> w1102
          tunnel: [w1139 w1150] -> w1113
          tunnel: [w1138 w1142] -> w1116
          tunnel: w1122 -> [_ w1149]
          tunnel: w1121 -> [_ w1148]
          tunnel: w1120 -> [_ _]
          tunnel: [_ w1145] -> w1114
          tunnel: [w1138 w1142] -> w1100
          tunnel: [w1138 w1141] -> w1099
          frame False {
            w1138 = "Skip" ("response")
          }
          frame True {
            w1155 = "UIdisplay" ("Process (\"\" - local)")
            n433 = call "get_parameter.vi"("Parameter"=T7[] ["derating_status"], "daemon reference in"=w1156) -> ("error out"=w1145:errorcluster, "response"=w1142:string, "daemon reference out"=w1150:refnum<k5>)  [unwired: 5 in, 2 out]
            n434 = call "Select_Table_Vaule.vi"("Boolean"=TRUE, "Vaule"=w1142, "Action"=w1149, "Table"=w1148) -> ("Result"=w1143:bool, "vaule"=w1147:string[])  [unwired: 6 in]
            n435 = Append True/False String(1:w1143, 2:"FAIL" ("真字符串"), 3:"PASS" ("真字符串")) -> (0:w1141:string)  [unwired: 1 in]
            n436 = Build Array (concatenate)(w1147, w1142, w1141) -> (w1154:string[])
            n437 = Flatten To XML(anything=w1154) -> (xml string=w1153:string)
            n438 = call "AMC Send Local Message.vi"("Process (\"\" - local)"=w1155, "Message Value"=w1153, "Message Name"=w1155) -> ()  [unwired: 7 in, 2 out]
          }
        }
        n439 = Unbundle By Name(w1104) -> ("Fail_resume_mode"=w1106:bool)
        n440 = property class="Bool (严格)"(reference=w1105) -> ("Value"=w1107:bool)  [unwired: 1 in, 2 out]
        n441 = Not(x=w1107) -> (.not. x?=w1108:bool)
        n442 = Or(x=w1106, y=w1108) -> (x .or. y?=w1110:bool)
        n443 = Select(t=TRUE, s=w1110, f=w1102) -> (s? t:f=w1101:bool)
        n444 = call <vilib>:"Space Constant.vi"() -> ("String"=w1125:string)
        n445 = Concatenate Strings(w1122, w1125, w1116) -> (w1124:string)
        n446 = Bundle By Name(cluster=w1127, "MAX.Max_check_derate_status_status"=w1102) -> (w1126:T3)
        n447 = Bundle By Name(cluster=w1115, "daemon reference"=w1113, "MAX.Check Derate Result"=w1100, "MAX_Status.Check Derate Result"=w1099) -> (w1112:T1)
        n448 = call "LogStatus.vi"("error in (no error)"=w1114, "last message"=w1129, "message"=w1124) -> ("error  out"=w1130:errorcluster)  [unwired: 8 in]
        n449 = case shown="No Error" w1114 {
          tunnel: w1101 -> [w1132 _]
          tunnel: [w1133 "Error"] -> w1118
          tunnel: [w1132 FALSE] -> w1117
          frame No Error {
            n450 = Select(t="Max_Get_Delta_Tmag_LSI_&_FISF", s=w1132, f="Finalization_NG_unit") -> (s? t:f=w1133:string)
          }
          frame Error {
          }
        }
        n451 = Not(x=w1117) -> (.not. x?=w1119:bool)
      }
      frame "Max_Get_Delta_Tmag_LSI_&_FISF" {
        n452 = Unbundle By Name(w1178) -> ("Table"=w1187:string[][], "daemon reference"=w1195:refnum<k5>, "Config"=w1186:string[][])
        n453 = call "Select_Table_Vaule Enable_Disable.vi"("Action"=w1188, "Table"=w1187) -> ("Enable"=w1189:bool)  [unwired: 8 in, 1 out]
        n454 = case shown="False" w1189 {
          tunnel: w1195 -> [w1209 w1229]
          tunnel: [TRUE w1226] -> _
          tunnel: [w1209 w1228] -> w1175
          tunnel: [w1207 w1221] -> w1190
          tunnel: w1188 -> [_ w1223]
          tunnel: w1187 -> [_ w1227]
          tunnel: w1186 -> [_ _]
          tunnel: [_ w1216] -> w1185
          tunnel: [_ w1225] -> w1177
          tunnel: [_ w1217] -> w1179
          tunnel: [T9 {"LSI Delta in degC"="Skip", "FISF Delta in degc"="Skip", "LSI Tmag in degC"="Skip", "Fisf Tmag in degC"="Skip", "IIR Tmag in degC"="Skip"} w1215] -> w1176
          tunnel: [w1206 w1211] -> w1159
          frame False {
            w1207 = "Skip" ("response")
            n455 = Initialize Array(w1207, 6 ("维数大小")) -> (w1206:string[])
          }
          frame True {
            n456 = call "get_delta_tmag.vi"("daemon reference in"=w1229) -> ("error out"=w1225:errorcluster, "Tmag Data"=w1216:T8, "response"=w1221:string, "daemon reference out"=w1228:refnum<k5>)  [unwired: 6 in, 1 out]
            n457 = Build Array (concatenate)(w1223, string[] ["Max_LSI_Delta_in_degC_after_tune", "Max_FISF_Delta_in_degC_after_tune", "Max_LSI_Tmag_in_degC_after_tune", "Max_Fisf_Tmag_in_degC_after_tune", "Max_IIR_Tmag_in_degC_after_tune"]) -> (w1219:string[])
            n458 = Cluster To Array(cluster=w1216) -> (array=w1224:dbl[])
            n459 = Number To Fractional String(number=w1216) -> (F-format string=w1215:T9)  [unwired: 3 in]
            n460 = Number To Fractional String(number=w1224) -> (F-format string=w1220:string[])  [unwired: 3 in]
            n461 = Build Array (concatenate)(w1221, w1220) -> (w1218:string[])
            n462 = for {
              tunnel: w1227 -> [w1235]
              tunnel: [w1231] -> w1226
              tunnel: w1219 -> [w1233] mode=indexing
              tunnel: w1218 -> [w1232] mode=indexing
              tunnel: [w1231] -> w1217 mode=indexing
              tunnel: [w1230] -> w1212 mode=indexing
              w1240 = "UIdisplay" ("Process (\"\" - local)")
              n463 = call "Select_Table_Vaule.vi"("Vaule"=w1232, "Action"=w1233, "Table"=w1235) -> ("Result"=w1231:bool, "vaule"=w1234:string[])  [unwired: 7 in]
              n464 = Append True/False String(1:w1231, 2:"FAIL" ("真字符串"), 3:"PASS" ("真字符串")) -> (0:w1230:string)  [unwired: 1 in]
              n465 = Build Array (concatenate)(w1234, w1232, w1230) -> (w1239:string[])
              n466 = Flatten To XML(anything=w1239) -> (xml string=w1238:string)
              n467 = call "AMC Send Local Message.vi"("Process (\"\" - local)"=w1240, "Message Value"=w1238, "Message Name"=w1240) -> ()  [unwired: 7 in, 2 out]
            }
            n468 = Delete From Array(array=w1212, length=1 ("长度"), index=0 ("索引")) -> (array with subset deleted=w1211:string[])  [unwired: 1 out]
          }
        }
        n469 = Unbundle By Name(w1163) -> ("MES bool"=w1167:refnum<vi>)
        n470 = call "HD_Config.vi"("Step"=enum16{"Initial", "Write", "Read"}."Read") -> ("HD Config out"=w1166:T5)  [unwired: 9 in, 1 out]
        n471 = Unbundle By Name(w1166) -> ("Fail_resume_mode"=w1168:bool)
        n472 = property class="Bool (严格)"(reference=w1167) -> ("Value"=w1169:bool)  [unwired: 1 in, 2 out]
        n473 = call <vilib>:"Space Constant.vi"() -> ("String"=w1192:string)
        n474 = Not(x=w1169) -> (.not. x?=w1170:bool)
        n475 = Concatenate Strings(w1188, w1192, w1190) -> (w1191:string)
        n476 = Or(x=w1168, y=w1170) -> (x .or. y?=w1171:bool)
        n477 = Delete From Array(array=w1179, length=1 ("长度"), index=0 ("索引")) -> (array with subset deleted=w1174:bool[])  [unwired: 1 out]
        n478 = Unbundle By Name(w1176) -> ("FISF Delta in degc"=w1160:string)
        n479 = Index Array(array=w1159, index=1 ("索引")) -> (element=w1157:string)
        n480 = Index Array(array=w1174, index=1 ("索引")) -> (element=w1162:bool)
        n481 = And Array Elements(Boolean array=w1174) -> ()  [unwired: 1 out]
        n482 = Bundle By Name(cluster=w1194, "MAX.Average_Tmag_Data_after_tune_status"=w1174, "MAX.Delta_Tmag_after_tune"=w1185) -> (w1193:T3)
        n483 = Bundle By Name(cluster=w1178, "MAX_Status.Delta Tmag FISF"=w1157, "MAX.Delta Tmag FISF"=w1160, "daemon reference"=w1175) -> (w1172:T1)
        n484 = Select(t=TRUE, s=w1171, f=w1162) -> (s? t:f=w1161:bool)
        n485 = call "LogStatus.vi"("error in (no error)"=w1177, "last message"=w1196, "message"=w1191) -> ("error  out"=w1197:errorcluster)  [unwired: 8 in]
        n486 = case shown="No Error" w1177 {
          tunnel: [w1199 FALSE] -> w1184
          tunnel: [w1200 "Error"] -> w1183
          tunnel: w1161 -> [w1199 _]
          frame No Error {
            n487 = Select(t="Max_Get_Hot_Bemf_in_mV", s=w1199, f="Finalization_NG_unit") -> (s? t:f=w1200:string)
          }
          frame Error {
          }
        }
        n488 = Not(x=w1184) -> (.not. x?=w1182:bool)
      }
      frame "Max_Get_Hot_Bemf_in_mV" {
        n489 = Unbundle By Name(w1246) -> ("Table"=w1252:string[][], "daemon reference"=w1260:refnum<k5>, "Config"=w1251:string[][])
        n490 = call "Select_Table_Vaule Enable_Disable.vi"("Action"=w1253, "Table"=w1252) -> ("Enable"=w1254:bool)  [unwired: 8 in, 1 out]
        n491 = case shown="False" w1254 {
          tunnel: w1260 -> [w1267 w1285]
          tunnel: [TRUE w1275] -> _
          tunnel: [w1267 w1279] -> w1244
          tunnel: [w1266 w1269] -> w1255
          tunnel: w1253 -> [_ w1278]
          tunnel: w1252 -> [_ w1277]
          tunnel: w1251 -> [_ _]
          tunnel: [_ w1272] -> w1249
          tunnel: [_ w1271] -> w1245
          tunnel: [w1266 w1270] -> w1241
          tunnel: [w1266 w1269] -> w1242
          frame False {
            w1266 = "Skip" ("response")
          }
          frame True {
            w1284 = "UIdisplay" ("Process (\"\" - local)")
            n492 = call "get_parameter.vi"("Parameter"=T7[] ["fisf_measured_bemf"], "daemon reference in"=w1285) -> ("error out"=w1271:errorcluster, "response"=w1269:string, "values"=w1273:dbl[], "daemon reference out"=w1279:refnum<k5>)  [unwired: 5 in, 1 out]
            n493 = call "Select_Table_Vaule.vi"("Vaule"=w1269, "Action"=w1278, "Table"=w1277) -> ("Result"=w1275:bool, "vaule"=w1276:string[])  [unwired: 7 in]
            n494 = Index Array(array=w1273) -> (element=w1272:dbl)  [unwired: 1 in]
            n495 = Append True/False String(1:w1275, 2:"FAIL" ("真字符串"), 3:"PASS" ("真字符串")) -> (0:w1270:string)  [unwired: 1 in]
            n496 = Build Array (concatenate)(w1276, w1269, w1270) -> (w1283:string[])
            n497 = Flatten To XML(anything=w1283) -> (xml string=w1282:string)
            n498 = call "AMC Send Local Message.vi"("Process (\"\" - local)"=w1284, "Message Value"=w1282, "Message Name"=w1284) -> ()  [unwired: 7 in, 2 out]
          }
        }
        n499 = call <vilib>:"Space Constant.vi"() -> ("String"=w1257:string)
        n500 = Concatenate Strings(w1253, w1257, w1255) -> (w1256:string)
        n501 = Bundle By Name(cluster=w1246, "daemon reference"=w1244, "MAX.Get Hot BEMF Result"=w1242, "MAX_Status.Get Hot BEMF Result"=w1241) -> (w1243:T1)
        n502 = Bundle By Name(cluster=w1259, "MAX.Hot Bemf in mV"=w1249) -> (w1258:T3)
        n503 = call "LogStatus.vi"("error in (no error)"=w1245, "last message"=w1261, "message"=w1256) -> ("error  out"=w1262:errorcluster)  [unwired: 8 in]
        n504 = case shown="Error" w1245 {
          tunnel: [_ TRUE] -> w1247
          tunnel: [_ "Error"] -> w1248
          frame No Error {
          }
          frame Error {
          }
        }
      }
      frame "Max_Stop_motor" {
        n505 = Unbundle By Name(w1292) -> ("Table"=w1297:string[][], "daemon reference"=w1302:refnum<k5>, "Config"=w1296:string[][])
        n506 = call "Select_Table_Vaule Enable_Disable.vi"("Action"=w1298, "Table"=w1297) -> ("Enable"=w1299:bool)  [unwired: 8 in, 1 out]
        n507 = case shown="True" w1299 {
          tunnel: w1302 -> [w1313 w1329]
          tunnel: [TRUE w1319] -> _
          tunnel: [w1313 w1323] -> w1290
          tunnel: ["" ("response") w1317] -> w1294
          tunnel: w1298 -> [_ w1322]
          tunnel: w1297 -> [_ w1321]
          tunnel: w1296 -> [_ _]
          tunnel: [_ w1318] -> w1291
          tunnel: [_ w1317] -> _
          tunnel: [_ w1316] -> _
          tunnel: [_ w1315] -> _
          frame False {
          }
          frame True {
            w1315 = "STOP" ("Power Mode")
            w1328 = "UIdisplay" ("Process (\"\" - local)")
            n508 = call "drive_motor.vi"("Power Mode"=w1315, "daemon reference in"=w1329) -> ("error out"=w1318:errorcluster, "response"=w1317:string, "daemon reference out"=w1323:refnum<k5>)  [unwired: 6 in, 1 out]
            n509 = call "Select_Table_Vaule.vi"("Vaule"=w1317, "Action"=w1322, "Table"=w1321) -> ("Result"=w1319:bool, "vaule"=w1320:string[])  [unwired: 7 in]
            n510 = call "时间延迟"("error in (no error)"=w1318) -> ()  [unwired: 10 in, 1 out]
            n511 = Append True/False String(1:w1319, 2:"FAIL" ("真字符串"), 3:"PASS" ("真字符串")) -> (0:w1316:string)  [unwired: 1 in]
            n512 = Build Array (concatenate)(w1320, w1317, w1316) -> (w1327:string[])
            n513 = Flatten To XML(anything=w1327) -> (xml string=w1326:string)
            n514 = call "AMC Send Local Message.vi"("Process (\"\" - local)"=w1328, "Message Value"=w1326, "Message Name"=w1328) -> ()  [unwired: 7 in, 2 out]
          }
        }
        n515 = Unbundle By Name(w1288) -> ("GRR"=w1286:bool)
        n516 = call <vilib>:"Space Constant.vi"() -> ("String"=w1301:string)
        n517 = Concatenate Strings(w1298, w1301, w1294) -> (w1300:string)
        n518 = Bundle By Name(cluster=w1292, "daemon reference"=w1290) -> (w1289:T1)
        n519 = call "LogStatus.vi"("error in (no error)"=w1291, "last message"=w1303, "message"=w1300) -> ("error  out"=w1304:errorcluster)  [unwired: 8 in]
        n520 = case shown="No Error" w1291 {
          tunnel: [w1306 TRUE] -> w1295
          tunnel: [w1308 "Error"] -> w1287
          tunnel: w1286 -> [w1306 _]
          frame No Error {
            n521 = Select(t="Finalization_NG_unit", s=w1306, f="Max_Get_DDM_Pressure") -> (s? t:f=w1308:string)
          }
          frame Error {
          }
        }
      }
      frame "Max_Get_DDM_Pressure" {
        n522 = Unbundle By Name(w1333) -> ("Table"=w1339:string[][], "daemon reference"=w1347:refnum<k5>, "Config"=w1338:string[][])
        n523 = call "Select_Table_Vaule Enable_Disable.vi"("Action"=w1340, "Table"=w1339) -> ("Enable"=w1341:bool)  [unwired: 8 in, 1 out]
        n524 = case shown="True" w1341 {
          tunnel: w1347 -> [w1354 w1374]
          tunnel: [TRUE w1364] -> _
          tunnel: [w1354 w1368] -> w1332
          tunnel: ["" ("response") w1356] -> w1342
          tunnel: w1340 -> [_ w1367]
          tunnel: w1339 -> [_ w1366]
          tunnel: w1338 -> [_ _]
          tunnel: [_ w1358] -> w1336
          tunnel: [_ w1359] -> w1330
          tunnel: [_ w1357] -> _
          tunnel: [_ w1356] -> _
          frame False {
          }
          frame True {
            w1373 = "UIdisplay" ("Process (\"\" - local)")
            n525 = call "get_parameter.vi"("Parameter"=T7[] ["pressure"], "daemon reference in"=w1374) -> ("error out"=w1359:errorcluster, "values"=w1362:dbl[], "daemon reference out"=w1368:refnum<k5>)  [unwired: 5 in, 2 out]
            n526 = Index Array(array=w1362) -> (element=w1361:dbl)  [unwired: 1 in]
            n527 = Divide(x=w1361, y=1000.0) -> (x/y=w1358:dbl)
            n528 = Number To Fractional String(number=w1358) -> (F-format string=w1356:string)  [unwired: 3 in]
            n529 = call "Select_Table_Vaule.vi"("Vaule"=w1356, "Action"=w1367, "Table"=w1366) -> ("Result"=w1364:bool, "vaule"=w1365:string[])  [unwired: 7 in]
            n530 = Append True/False String(1:w1364, 2:"FAIL" ("真字符串"), 3:"PASS" ("真字符串")) -> (0:w1357:string)  [unwired: 1 in]
            n531 = Build Array (concatenate)(w1365, w1356, w1357) -> (w1372:string[])
            n532 = Flatten To XML(anything=w1372) -> (xml string=w1371:string)
            n533 = call "AMC Send Local Message.vi"("Process (\"\" - local)"=w1373, "Message Value"=w1371, "Message Name"=w1373) -> ()  [unwired: 7 in, 2 out]
          }
        }
        n534 = call <vilib>:"Space Constant.vi"() -> ("String"=w1344:string)
        n535 = Concatenate Strings(w1340, w1344, w1342) -> (w1343:string)
        n536 = Bundle By Name(cluster=w1333, "daemon reference"=w1332) -> (w1331:T1)
        n537 = Bundle By Name(cluster=w1346, "MAX.DDM_Pressure"=w1336) -> (w1345:T3)
        n538 = call "LogStatus.vi"("error in (no error)"=w1330, "last message"=w1348, "message"=w1343) -> ("error  out"=w1349:errorcluster)  [unwired: 8 in]
        n539 = case shown="Error" w1330 {
          tunnel: [_ TRUE] -> w1334
          tunnel: [_ "Error"] -> w1335
          frame No Error {
          }
          frame Error {
          }
        }
      }
      frame "Max_Calculate_the_delta_pressure" {
        n540 = Unbundle By Name(w1410) -> ("MAX.DDM_Pressure"=w1403:dbl)
        n541 = Unbundle By Name(w1383) -> ("Table"=w1382:string[][])
        n542 = call "HD_Config.vi"("Step"=enum16{"Initial", "Write", "Read"}."Read") -> ("HD Config out"=w1396:T5)  [unwired: 9 in, 1 out]
        n543 = Unbundle By Name(w1396) -> ("Lefoo.COM"=w1395:refnum<visa-resource-name>)
        n544 = call "Select_Table_Vaule Enable_Disable.vi"("Action"="Airwatts_Tune", "Table"=w1382) -> ()  [unwired: 8 in, 2 out]
        n545 = call "Lefoo Atmospheric pressure.vi"("VISA resource name"=w1395) -> ("Atmospheric pressure"=w1393:dbl)  [unwired: 8 in, 2 out]
        n546 = Subtract(x=w1403, y=w1393) -> (x-y=w1402:dbl)
        n547 = call "Select_Table_Vaule Enable_Disable.vi"("Action"=w1404, "Table"=w1382) -> ("Enable"=w1405:bool)  [unwired: 8 in, 1 out]
        n548 = case shown="False" w1405 {
          tunnel: [TRUE w1420] -> w1379
          tunnel: [w1415 w1418] -> w1406
          tunnel: w1404 -> [_ w1423]
          tunnel: w1382 -> [_ w1422]
          tunnel: [_ w1419] -> w1394
          tunnel: w1402 -> [_ w1419]
          tunnel: [w1415 w1418] -> w1377
          tunnel: [w1415 w1417] -> w1376
          frame False {
            w1415 = "Skip" ("response")
          }
          frame True {
            w1428 = "UIdisplay" ("Process (\"\" - local)")
            n549 = Number To Fractional String(number=w1419) -> (F-format string=w1418:string)  [unwired: 3 in]
            n550 = call "Select_Table_Vaule.vi"("Vaule"=w1418, "Action"=w1423, "Table"=w1422) -> ("Result"=w1420:bool, "vaule"=w1421:string[])  [unwired: 7 in]
            n551 = Append True/False String(1:w1420, 2:"FAIL" ("真字符串"), 3:"PASS" ("真字符串")) -> (0:w1417:string)  [unwired: 1 in]
            n552 = Build Array (concatenate)(w1421, w1418, w1417) -> (w1427:string[])
            n553 = Flatten To XML(anything=w1427) -> (xml string=w1426:string)
            n554 = call "AMC Send Local Message.vi"("Process (\"\" - local)"=w1428, "Message Value"=w1426, "Message Name"=w1428) -> ()  [unwired: 7 in, 2 out]
          }
        }
        n555 = call <vilib>:"Space Constant.vi"() -> ("String"=w1408:string)
        n556 = Concatenate Strings(w1404, w1408, w1406) -> (w1407:string)
        n557 = Unbundle By Name(w1385) -> ("MES bool"=w1388:refnum<vi>)
        n558 = call "HD_Config.vi"("Step"=enum16{"Initial", "Write", "Read"}."Read") -> ("HD Config out"=w1387:T5)  [unwired: 9 in, 1 out]
        n559 = Unbundle By Name(w1387) -> ("Fail_resume_mode"=w1389:bool)
        n560 = property class="Bool (严格)"(reference=w1388) -> ("Value"=w1390:bool)  [unwired: 1 in, 2 out]
        n561 = Not(x=w1390) -> (.not. x?=w1391:bool)
        n562 = Or(x=w1389, y=w1391) -> (x .or. y?=w1380:bool)
        n563 = Bundle By Name(cluster=w1383, "MAX_Status.Calculate delta Pressure"=w1376, "MAX.Calculate delta Pressure"=w1377) -> (w1392:T1)
        n564 = Select(t=TRUE, s=w1380, f=w1379) -> (s? t:f=w1378:bool)
        n565 = call "LogStatus.vi"("error in (no error)"=w1413, "last message"=w1411, "message"=w1407) -> ("error  out"=w1412:errorcluster)  [unwired: 8 in]
        n566 = Select(t="Max_Save_Calibration", s=w1378, f="Finalization_NG_unit") -> (s? t:f=w1375:string)
        n567 = Bundle By Name(cluster=w1410, "MAX.Delta_Pressure"=w1394, "MAX.Delta_Pressure_status"=w1379) -> (w1409:T3)
        n568 = Select(t="Max_Get_Cold_Bemf_in_mV", s=w1380, f=w1375) -> ()  [unwired: 1 out]
        n569 = Not(x=w1378) -> (.not. x?=w1399:bool)
      }
      frame "Max_Save_Calibration" {
        n570 = Unbundle By Name(w1442) -> ("Table"=w1449:string[][], "daemon reference"=w1454:refnum<k5>, "Config"=w1448:string[][])
        n571 = Unbundle By Name(w1430) -> ("MES bool"=w1435:refnum<vi>)
        n572 = call "HD_Config.vi"("Step"=enum16{"Initial", "Write", "Read"}."Read") -> ("HD Config out"=w1436:T5)  [unwired: 9 in, 1 out]
        n573 = Unbundle By Name(w1436) -> ("Fail_resume_mode"=w1434:bool)
        n574 = property class="Bool (严格)"(reference=w1435) -> ("Value"=w1433:bool)  [unwired: 1 in, 2 out]
        n575 = call "Select_Table_Vaule Enable_Disable.vi"("Action"=w1450, "Table"=w1449) -> ("Enable"=w1451:bool)  [unwired: 8 in, 1 out]
        n576 = Not(x=w1433) -> (.not. x?=w1432:bool)
        n577 = Or(x=w1434, y=w1432) -> (x .or. y?=w1429:bool)
        n578 = case shown="False" w1451 {
          tunnel: w1454 -> [w1461 w1475]
          tunnel: [TRUE w1467] -> _
          tunnel: [w1461 w1471] -> w1440
          tunnel: [w1460 w1465] -> w1444
          tunnel: w1450 -> [_ w1470]
          tunnel: w1449 -> [_ w1469]
          tunnel: w1448 -> [_ _]
          tunnel: [_ w1466] -> w1441
          tunnel: [w1460 w1465] -> w1438
          tunnel: [w1460 w1464] -> w1437
          tunnel: w1429 -> [_ w1463]
          frame False {
            w1460 = "Skip" ("response")
          }
          frame True {
            w1474 = "UIdisplay" ("Process (\"\" - local)")
            n579 = case shown="True" w1463 {
              tunnel: w1475 -> [w1484 w1486]
              tunnel: [w1483 w1486] -> w1471
              tunnel: [w1482 _] -> w1466
              tunnel: [w1481 "Skip" ("response")] -> w1465
              frame False {
                n580 = call "finalise_calibration.vi"("daemon reference in"=w1484) -> ("error out"=w1482:errorcluster, "response"=w1481:string, "daemon reference out"=w1483:refnum<k5>)  [unwired: 7 in, 1 out]
                n581 = call "时间延迟2"("error in (no error)"=w1482) -> ()  [unwired: 10 in, 1 out]
              }
              frame True {
              }
            }
            n582 = call "Select_Table_Vaule.vi"("Vaule"=w1465, "Action"=w1470, "Table"=w1469) -> ("Result"=w1467:bool, "vaule"=w1468:string[])  [unwired: 7 in]
            n583 = case shown="True" w1463 {
              tunnel: w1467 -> [w1477 _]
              tunnel: [w1476 "Skip" ("response")] -> w1464
              frame False {
                n584 = Append True/False String(1:w1477, 2:"FAIL" ("真字符串"), 3:"PASS" ("真字符串")) -> (0:w1476:string)  [unwired: 1 in]
              }
              frame True {
              }
            }
            n585 = Build Array (concatenate)(w1468, w1465, w1464) -> (w1473:string[])
            n586 = Flatten To XML(anything=w1473) -> (xml string=w1472:string)
            n587 = call "AMC Send Local Message.vi"("Process (\"\" - local)"=w1474, "Message Value"=w1472, "Message Name"=w1474) -> ()  [unwired: 7 in, 2 out]
          }
        }
        n588 = call <vilib>:"Space Constant.vi"() -> ("String"=w1453:string)
        n589 = Concatenate Strings(w1450, w1453, w1444) -> (w1452:string)
        n590 = Bundle By Name(cluster=w1442, "daemon reference"=w1440, "MAX.Finalise Calibration"=w1438, "MAX_Status.Finalise Calibration"=w1437) -> (w1439:T1)
        n591 = call "LogStatus.vi"("error in (no error)"=w1441, "last message"=w1455, "message"=w1452) -> ("error  out"=w1456:errorcluster)  [unwired: 8 in]
        n592 = case shown="Error" w1441 {
          tunnel: [_ TRUE] -> w1445
          tunnel: [_ "Error"] -> w1446
          frame No Error {
          }
          frame Error {
          }
        }
      }
      frame "Max_Get_Cold_Bemf_in_mV" {
        n593 = Unbundle By Name(w1490) -> ("Table"=w1496:string[][], "daemon reference"=w1504:refnum<k5>, "Config"=w1495:string[][])
        n594 = call "Select_Table_Vaule Enable_Disable.vi"("Action"=w1497, "Table"=w1496) -> ("Enable"=w1498:bool)  [unwired: 8 in, 1 out]
        n595 = case shown="True" w1498 {
          tunnel: w1504 -> [w1511 w1529]
          tunnel: [TRUE w1519] -> _
          tunnel: [w1511 w1523] -> w1488
          tunnel: ["" ("response") w1514] -> w1499
          tunnel: w1497 -> [_ w1522]
          tunnel: w1496 -> [_ w1521]
          tunnel: w1495 -> [_ _]
          tunnel: [_ w1516] -> w1493
          tunnel: [_ w1515] -> w1489
          tunnel: [_ w1514] -> _
          tunnel: [_ w1513] -> _
          frame False {
          }
          frame True {
            w1528 = "UIdisplay" ("Process (\"\" - local)")
            n596 = call "get_calibration.vi"("Calibration"=T10[] ["eol_cold_bemf_fisf"], "daemon reference in"=w1529) -> ("error out"=w1515:errorcluster, "response"=w1514:string, "values"=w1517:dbl[], "daemon reference out"=w1523:refnum<k5>)  [unwired: 5 in, 1 out]
            n597 = call "Select_Table_Vaule.vi"("Vaule"=w1514, "Action"=w1522, "Table"=w1521) -> ("Result"=w1519:bool, "vaule"=w1520:string[])  [unwired: 7 in]
            n598 = Index Array(array=w1517) -> (element=w1516:dbl)  [unwired: 1 in]
            n599 = Append True/False String(1:w1519, 2:"FAIL" ("真字符串"), 3:"PASS" ("真字符串")) -> (0:w1513:string)  [unwired: 1 in]
            n600 = Build Array (concatenate)(w1520, w1514, w1513) -> (w1527:string[])
            n601 = Flatten To XML(anything=w1527) -> (xml string=w1526:string)
            n602 = call "AMC Send Local Message.vi"("Process (\"\" - local)"=w1528, "Message Value"=w1526, "Message Name"=w1528) -> ()  [unwired: 7 in, 2 out]
          }
        }
        n603 = call <vilib>:"Space Constant.vi"() -> ("String"=w1501:string)
        n604 = Concatenate Strings(w1497, w1501, w1499) -> (w1500:string)
        n605 = Bundle By Name(cluster=w1490, "daemon reference"=w1488) -> (w1487:T1)
        n606 = Bundle By Name(cluster=w1503, "MAX.Cold Bemf in mV"=w1493) -> (w1502:T3)
        n607 = call "LogStatus.vi"("error in (no error)"=w1489, "last message"=w1505, "message"=w1500) -> ("error  out"=w1506:errorcluster)  [unwired: 8 in]
        n608 = case shown="No Error" w1489 {
          tunnel: [_ TRUE] -> w1491
          tunnel: [_ "Error"] -> w1492
          frame No Error {
          }
          frame Error {
          }
        }
      }
      frame "Max_Calculate_and_Check_delta_BEMF" {
        n609 = Unbundle By Name(w1560) -> ("MAX.Cold Bemf in mV"=w1553:dbl, "MAX.Hot Bemf in mV"=w1548:dbl)
        n610 = Unbundle By Name(w1544) -> ("Table"=w1546:string[][])
        n611 = Subtract(x=w1553, y=w1548) -> (x-y=w1552:dbl)
        n612 = call "Select_Table_Vaule Enable_Disable.vi"("Action"=w1554, "Table"=w1546) -> ("Enable"=w1555:bool)  [unwired: 8 in, 1 out]
        n613 = case shown="False" w1555 {
          tunnel: [TRUE w1571] -> w1533
          tunnel: [w1565 w1568] -> w1556
          tunnel: w1554 -> [_ w1574]
          tunnel: w1546 -> [_ w1573]
          tunnel: [_ w1569] -> w1545
          tunnel: w1552 -> [_ w1569]
          tunnel: [w1565 w1568] -> w1531
          tunnel: [w1565 w1567] -> w1530
          frame False {
            w1565 = "Skip" ("response")
          }
          frame True {
            w1579 = "UIdisplay" ("Process (\"\" - local)")
            n614 = Multiply(x=1000.0, y=w1569) -> ()  [unwired: 1 out]
            n615 = Number To Fractional String(number=w1569) -> (F-format string=w1568:string)  [unwired: 3 in]
            n616 = call "Select_Table_Vaule.vi"("Vaule"=w1568, "Action"=w1574, "Table"=w1573) -> ("Result"=w1571:bool, "vaule"=w1572:string[])  [unwired: 7 in]
            n617 = Append True/False String(1:w1571, 2:"FAIL" ("真字符串"), 3:"PASS" ("真字符串")) -> (0:w1567:string)  [unwired: 1 in]
            n618 = Build Array (concatenate)(w1572, w1568, w1567) -> (w1578:string[])
            n619 = Flatten To XML(anything=w1578) -> (xml string=w1577:string)
            n620 = call "AMC Send Local Message.vi"("Process (\"\" - local)"=w1579, "Message Value"=w1577, "Message Name"=w1579) -> ()  [unwired: 7 in, 2 out]
          }
        }
        n621 = call <vilib>:"Space Constant.vi"() -> ("String"=w1558:string)
        n622 = Unbundle By Name(w1534) -> ("MES bool"=w1539:refnum<vi>)
        n623 = Concatenate Strings(w1554, w1558, w1556) -> (w1557:string)
        n624 = call "HD_Config.vi"("Step"=enum16{"Initial", "Write", "Read"}."Read") -> ("HD Config out"=w1538:T5)  [unwired: 9 in, 1 out]
        n625 = Unbundle By Name(w1538) -> ("Fail_resume_mode"=w1540:bool)
        n626 = property class="Bool (严格)"(reference=w1539) -> ("Value"=w1541:bool)  [unwired: 1 in, 2 out]
        n627 = Not(x=w1541) -> (.not. x?=w1542:bool)
        n628 = Or(x=w1540, y=w1542) -> (x .or. y?=w1537:bool)
        n629 = Bundle By Name(cluster=w1544, "MAX.Calculate & Check Delta BEMF"=w1531, "MAX_Status.Calculate & Check Delta BEMF"=w1530) -> (w1543:T1)
        n630 = Select(t=TRUE, s=w1537, f=w1533) -> (s? t:f=w1532:bool)
        n631 = call "LogStatus.vi"("error in (no error)"=w1563, "last message"=w1561, "message"=w1557) -> ("error  out"=w1562:errorcluster)  [unwired: 8 in]
        n632 = Bundle By Name(cluster=w1560, "MAX.delta Bemf"=w1545, "MAX.delta Bemf_status"=w1533) -> (w1559:T3)
        n633 = Not(x=w1532) -> (.not. x?=w1549:bool)
        n634 = Select(t="Max_Get_AW_Calibration", s=w1532, f="Finalization_NG_unit") -> (s? t:f=w1547:string)
      }
      frame "Max_Get_AW_Calibration" {
        n635 = Unbundle By Name(w1613) -> ("MAX.AW_Finetune.delta_P_Setting"=w1604:dbl, "MAX.AW_Tune.delta_P_Setting"=w1603:dbl, "MAX.Cal_Tester_Parameter_status"=w1601:bool[])
        n636 = Unbundle By Name(w1597) -> ("Table"=w1599:string[][], "daemon reference"=w1598:refnum<k5>)  [unwired: 1 out]
        n637 = call "Select_Table_Vaule Enable_Disable.vi"("Action"=w1607, "Table"=w1599) -> ("Enable"=w1608:bool)  [unwired: 8 in, 1 out]
        n638 = Index Array(array=w1601, index=4) -> (element=w1602:bool)
        n639 = case shown="False" w1608 {
          tunnel: w1598 -> [w1623 w1645]
          tunnel: [TRUE w1629] -> w1583
          tunnel: [w1623 w1639] -> w1594
          tunnel: [w1622 w1627] -> w1609
          tunnel: w1607 -> [_ w1638]
          tunnel: w1599 -> [_ w1637]
          tunnel: w1604 -> [_ w1632]
          tunnel: w1603 -> [_ w1631]
          tunnel: [_ w1630] -> w1595
          tunnel: [_ w1633] -> w1596
          tunnel: w1602 -> [_ w1628]
          tunnel: [w1622 w1626] -> w1581
          tunnel: [w1622 w1625] -> w1580
          frame False {
            w1622 = "Skip" ("response")
          }
          frame True {
            w1644 = "UIdisplay" ("Process (\"\" - local)")
            n640 = call "get_aw_tune.vi"("Index"=u32 2, "daemon reference in"=w1645) -> ("error out"=w1633:errorcluster, "AW Tune Parameter"=w1634:T13, "response"=w1627:string, "daemon reference out"=w1639:refnum<k5>)  [unwired: 5 in, 1 out]
            n641 = Unbundle By Name(w1634) -> ("Offset power mW"=w1630:i64)
            n642 = case shown="False" w1628 {
              selector: w1628 -> [_ w1654]
              tunnel: w1632 -> [w1653 _]
              tunnel: w1631 -> [w1652 _]
              tunnel: w1630 -> [w1650 _]
              tunnel: [w1648 w1654] -> w1629
              frame False {
                n643 = To Long Integer(number=w1652) -> (32bit integer=w1649:i32)
                n644 = To Long Integer(number=w1653) -> (32bit integer=w1651:i32)
                n645 = Equal?(x=w1650, y=w1651) -> (x = y?=w1647:bool)
                n646 = Equal?(x=w1650, y=w1649) -> (x = y?=w1646:bool)
                n647 = Or(x=w1647, y=w1646) -> (x .or. y?=w1648:bool)
              }
              frame True {
              }
            }
            n648 = call "Select_Table_Vaule.vi"("Vaule"=w1627, "Action"=w1638, "Table"=w1637) -> ("vaule"=w1636:string[])  [unwired: 7 in, 1 out]
            n649 = Append True/False String(1:w1629, 2:"FAIL" ("真字符串"), 3:"PASS" ("真字符串")) -> (0:w1626:string)  [unwired: 1 in]
            n650 = Build Array (concatenate)(w1636, w1627, w1626) -> (w1643:string[])
            n651 = Flatten To XML(anything=w1643) -> (xml string=w1642:string)
            n652 = Number To Fractional String(number=w1630) -> (F-format string=w1625:string)  [unwired: 3 in]
            n653 = call "AMC Send Local Message.vi"("Process (\"\" - local)"=w1644, "Message Value"=w1642, "Message Name"=w1644) -> ()  [unwired: 7 in, 2 out]
          }
        }
        n654 = Unbundle By Name(w1584) -> ("MES bool"=w1589:refnum<vi>)
        n655 = call "HD_Config.vi"("Step"=enum16{"Initial", "Write", "Read"}."Read") -> ("HD Config out"=w1588:T5)  [unwired: 9 in, 1 out]
        n656 = Unbundle By Name(w1588) -> ("Fail_resume_mode"=w1590:bool)
        n657 = property class="Bool (严格)"(reference=w1589) -> ("Value"=w1591:bool)  [unwired: 1 in, 2 out]
        n658 = call <vilib>:"Space Constant.vi"() -> ("String"=w1611:string)
        n659 = Not(x=w1591) -> (.not. x?=w1592:bool)
        n660 = Or(x=w1590, y=w1592) -> (x .or. y?=w1587:bool)
        n661 = Concatenate Strings(w1607, w1611, w1609) -> (w1610:string)
        n662 = Select(t=TRUE, s=w1587, f=w1583) -> (s? t:f=w1582:bool)
        n663 = case shown="No Error" w1596 {
          tunnel: [w1619 "Error"] -> w1606
          tunnel: w1582 -> [w1618 _]
          frame No Error {
            n664 = Select(t="Task_Detect_Calibration", s=w1618, f="Finalization_NG_unit") -> (s? t:f=w1619:string)
          }
          frame Error {
          }
        }
        n665 = Bundle By Name(cluster=w1597, "MAX_Status.Delta P Airwatts Value"=w1581, "MAX.Delta P Airwatts Value"=w1580, "daemon reference"=w1594) -> (w1593:T1)
        n666 = call "LogStatus.vi"("error in (no error)"=w1596, "last message"=w1614, "message"=w1610) -> ("error  out"=w1615:errorcluster)  [unwired: 8 in]
        n667 = Bundle By Name(cluster=w1613, "MAX.delta p"=w1595) -> (w1612:T3)
      }
    }
    n668 = call "6-AlarmStatus.vi"("Step"=enum16{"Initial", "Write", "Read"}."Read") -> ("AlarmValue Out"=w18:bool[])  [unwired: 9 in, 1 out]
    n669 = call "Stop.vi"("Step"=enum16{"Initial", "Write", "Read"}."Read") -> ("Stop Out"=w26:bool)  [unwired: 9 in, 1 out]
    n670 = call "Exit.vi"("Step"=enum16{"Initial", "Write", "Read"}."Read" ("step")) -> ("Exit Out"=w25:bool)  [unwired: 9 in, 1 out]
    n671 = Or Array Elements(Boolean array=w18) -> (logical OR=w17:bool)
    n672 = Compound Arithmetic op=OR(w24, w26, w25, w17) -> (w23:bool)
    n673 = call "AMC Run Step.vi"("Message Queue In"=w44, "Message Name"=w32, "Message Value"=w30, "error in (no error)"=w39, "Mli/Sig"=FALSE) -> ("Message Queue Out"=w43:T4, "error out"=w38:errorcluster)  [unwired: 13 in]
  }
  "Message Queue Out" <- w6
  "error out" <- w5
  "Data" <- w10
  "Flow" <- w7
  "Data out" <- w1
